vi "CRYMultimeter.vi"(0 "Device In":u32, 1 "Signal Path":i32(ring) caption="信号通道" items=["Left", "Right"], 2 "Mode":i32(slide), 3 "Time(sec)":dbl=5.0 caption="时间(秒)" min=0.05 max=10.0 step=0.05 format="%.0p", 4 "Avg.Time(sec)":dbl=1.0 caption="平均时间(秒)" min=0.05 max=1000.0 step=0.05 format="%.0p", 7 "Calibration in":string, 8 "Lin/Exp":i32(slide), 9 "Hardware in":string, 10 "Manual":bool=TRUE, 11 "Execution control":T3={"interactive"=TRUE, "displayed"=TRUE, "in a seq"=FALSE}, 13 "Cancel":bool) -> (6 "VMax In":dbl=1.0 min=0.1 max=10.0 step=0.01 format="%.3f", 12 "Canceled?":bool, 14 "InputLevel Out":T2, 15 "dB":cluster{dbl, dbl}(slide)={-inf, 99.22598823705182} scale=-70.01029995663981..19.989700043360187, 16 "Channel In":u16, 17 "Record time out":dbl format="%.2f", 18 "Averages out":i32, 19 "Overload":bool)   [LabVIEW 2013]
uses:
  Typedef Control/CRYData Cluster.ctl
  Typedef Control/CRYHardware Channel Info.ctl
  <vilib>/Analysis/baseanly.llb/Mean (DBL).vi
  <vilib>/Analysis/baseanly.llb/Real Dot Product.vi
  SubVI/CRYMisc vis settings global.vi
  Calibration/SubVI/CRYCal Global.vi
  Limits/CRYLimit edit global.vi
  CRYMainGlobal.vi
  Task Sequence/CRYProject Run Control Global.vi
  <vilib>/Analysis/NI_AALPro.lvlib
  <vilib>/Analysis/NI_AALBase.lvlib
  CRYSound.dll
panel:
  out "WWWW 2":dbl[](array[numeric])
  out "WWWW":dbl[](array[numeric])
  out "Corr Curve":T1={"Name"="", "Curve"=[], "X data"=1, "Y data"=1, "Z data"=1, "X axis"=0, "Y axis"=1, "Z axis"=1, "X unit"="Hz", "Y unit"="", "Z unit"="deg.", "X dB ref"=1.0, "Y dB ref"=1.0, "Z dB ref"=1.0, "single val"=FALSE, "protected"=FALSE, "display X"=TRUE, "display Y"=TRUE, "display Z"=TRUE, "Test Info"="", "Step No."=0, "Plot Settings"={"Color"=0, "Interpolation"=0, "Point Style"=0, "Line Style"=0, "Point Color"=0, "Line Width"=0, "Bar Plot Style"=0, "Fill To"=0}, "AutoProtect"=FALSE} {"Z data" items=["dB", "Lin"]; "X data" items=["dB", "Lin"]; "Y data" items=["dB", "Lin"]; "Z dB ref" format="%.1f"; "Z axis" items=["Log", "Lin"]; "X dB ref" format="%.1f"; "X axis" items=["Log", "Lin"]; "Y axis" items=["Log", "Lin"]; "Y dB ref" format="%.1f"; "Curve"."z" format="%.2f"; "Curve"."y" format="%.2f"; "Curve"."x" format="%.2f"}
  out "Waveform Graph":dbl[][](graph)
  out "y(n-1)":dbl
  in  "Buf Cnt":i32
  in  "isMain":bool
  in  "Rcv Idx":u16
  in  "start_flg":u8
  in  "ASIO_Inited":bool
  out "Asio OCI":u32
  in  "Remain Data":i32[](array[numeric])
  in  "Device Name":string
  in  "Audio Driver":u16
  out "Load Test":bool
  out "Set Configure":bool
  out "Configure Data":string
  out "Lower Str":bool
  out "Upper Str":bool
  out "initialized array":i32[](array[numeric])
  out "Menu":bool=TRUE
  out "StateOut":bool=TRUE
  out "VI nID":i32
  out "Title nID":i32
  out "User Avg.Time(sec)":dbl
  out "return type":u32
  out "multimeter setup Out":string="%#_6p"
  out "nBufferUse":u32
  out "RealTime":u32
  out "OverHead":u8
  in  "taskID":u32
  out "InputLevel":dbl caption="输入电平" step=1.0 format="%.3p"
  in  "Continue":bool
  out "AveString":bool
  in  "Start":bool
  in  "Lower limit":cluster{dbl, dbl}(slide)={100.0, 4.285714285714286} caption="Upper limit" scale=-70.01029995663981..19.989700043360187
  out "unit 2":string="dB"
  out "Averaging":bool caption="平均"
  out "Input":bool caption="输入"
  in  "Apply Correction":bool caption="修正"
  in  "Weighting":i32(ring) caption="加权" items=["None", "A", "B", "C"]
  out "Elapsed Time":dbl=50.0 caption="经过时间" min=0.05 max=100000.0 step=0.05 format="%.2p"
  in  "Time Weighting":i32(ring) caption="时间计权" items=["Fast", "Slow", "User"]
  in  "Level":i32(slide) caption="weighting"
  in  "Bits":u32=16
  in  "Sampling rate":u32=44100
  in  "Channels":u8=2
  in  "OK":bool
  in  "Limits On":bool caption="显示上下限"
  out "Buffer Use %":i32
  out "Verdict":bool=TRUE
  in  "AC/DC":i32(slide)
  out "dB ref.":dbl=1.0 format="%.2f"
  out "Sens":dbl=1.0 format="%.2f"
  out "unit":string="V"
  in  "close at end":bool
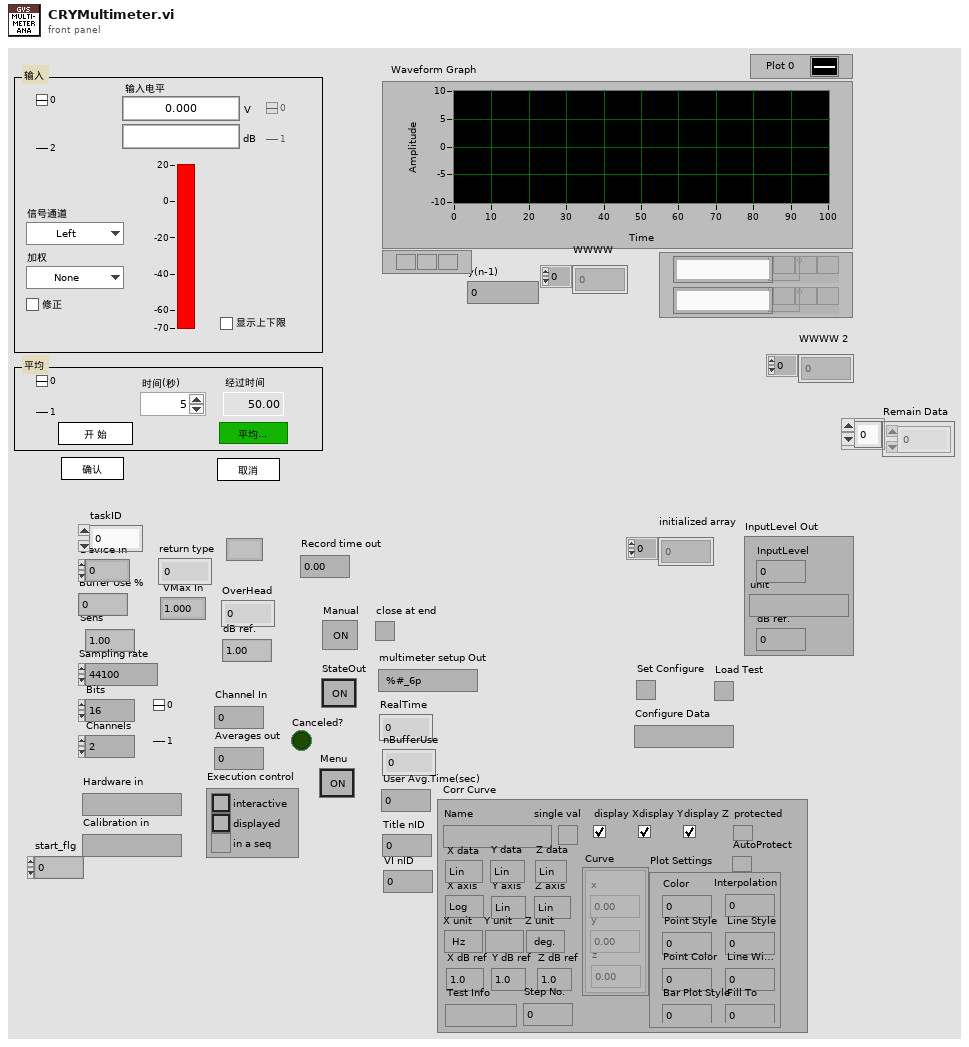
[diagram p1: front panel]
types:
  T1 = typedef "CRYData Cluster.ctl" = cluster{"Name":string, "Curve":cluster{"x":dbl, "y":dbl, "z":dbl}[], "X data":u16, "Y data":u16, "Z data":u16, "X axis":u16, "Y axis":u16, "Z axis":u16, "X unit":string, "Y unit":string, "Z unit":string, "X dB ref":dbl, "Y dB ref":dbl, "Z dB ref":dbl, "single val":bool, "protected":bool, "display X":bool, "display Y":bool, "display Z":bool, "Test Info":string, "Step No.":i32, "Plot Settings":cluster{"Color":u32, "Interpolation":u8, "Point Style":u8, "Line Style":u8, "Point Color":u32, "Line Width":u8, "Bar Plot Style":u8, "Fill To":i16}, "AutoProtect":bool}
  T2 = cluster{"InputLevel":dbl, "unit":string, "dB ref.":dbl}
  T3 = cluster{"interactive":bool, "displayed":bool, "in a seq":bool}
  T4 = cluster{"Start":bool, "Continue":bool, "OK":bool, "Cancel":bool, "Mode":i32, "Level":i32, "Channel":i32, "Weighting":i32, "Apply Correction":bool, "Limits On":bool, "Lin/Exp":i32, "Time Weighting":i32, "Time(sec)":dbl, "Avg.Time(sec)":dbl}
  T5 = typedef "CRYCalibration All Cluster.ctl" = cluster{"Calibration 2D":T6[], "Help":string, "Tab Value":i32, "Input Signal Type":string, "Output Signal Type":string}
  T6 = typedef "CRYCalibration 2DCluster.ctl" = cluster{"Calibration":T7, "Corr Curve":T1, "EQ Curve":T1, "Sens Curve":T1}
  T7 = typedef "CRYCalibration Cluster.ctl" = cluster{"Calibration Step Name":string, "Device":string, "Correction Curve Name":string, "Equalization Curve Name":string, "Sensitivity Curve Name":string, "Corr Folder and File":string, "EQ Folder and File":string, "Sens Folder and File":string, "Corr Step size":u16, "EQ Step size":u16, "Input":bool, "Last Cal Date (sec)":timestamp, "Cha Name":string, "Corr Curve Found":bool, "EQ Curve Found":bool, "Sens Curve Found":bool, "Signal Type":string, "Calibrated Device":string, "Hz":u32}
  T8 = typedef "CRYMultimeter.ctl" = cluster{"Ave/Max/Min":i32, "Level":i32, "Channel":i32, "Signal Type":string, "Weighting":string, "Applay Correction":bool, "lin/exp avg":u16, "rec time (sec)":dbl, "Average Time (Sec)":dbl, "Lin Display Prefs":string, "dB Display Prefs":string, "Time Weighting":u16, "Display":u16}
  T9 = typedef "CRYHardware Channel Info.ctl" = cluster{"ID":i32, "Name":string, "Digital":bool, "Input":bool, "Device Name":string, "Hardware Ch ID":u8, "Vmax (V)":dbl, "Latency (samples)":dbl, "Sampling Rate (Hz)":u32, "Bit Depth":u32, "Anti-aliasing Factor (%fs)":sgl, "DAQmx Channel":tag, "term config":i32, "Coupling":i32, "IEPE en":bool, "ASIOChannel Name":string, "Audio Driver":u16, "ASIOChannel Index":u8}
  T10 = typedef "LVPositionTypeDef.ctl" = cluster{"Left":i32, "Top":i32}
  T11 = cluster{"acquire":bool, "halt acq":bool, "n avgd":i32, "avg. complete":i32, "buffers":i32, "cal factor1":dbl, "cal factor2":dbl, "cal factor3":dbl, "update":bool, "Avg.weighting":dbl[], "Time Weighting":i32, "Avg.Time(sec)":dbl, "Continue":bool, "Mode":i32, "Level":i32, "Channel":i32, "rms max":dbl, "rms min":dbl, "avg. hold":dbl, "update ch":bool, "peak max":dbl, "peak min":dbl, "Weighting Curve":T1}
  T12 = cluster{"Start":bool, "Continue":bool, "OK":bool, "Cancel":bool, "Mode":i32, "Level":i32, "Signal Path":i32, "Weighting":i32, "Apply Correction":bool, "Limits On":bool, "Lin/Exp":i32, "Time Weighting":i32, "Time(sec)":dbl, "Avg.Time(sec)":dbl}
  T13 = cluster{"Rcv Idx":i32, "Chn Idx":i32, "Data":i32[], "bufCount":i32}[]
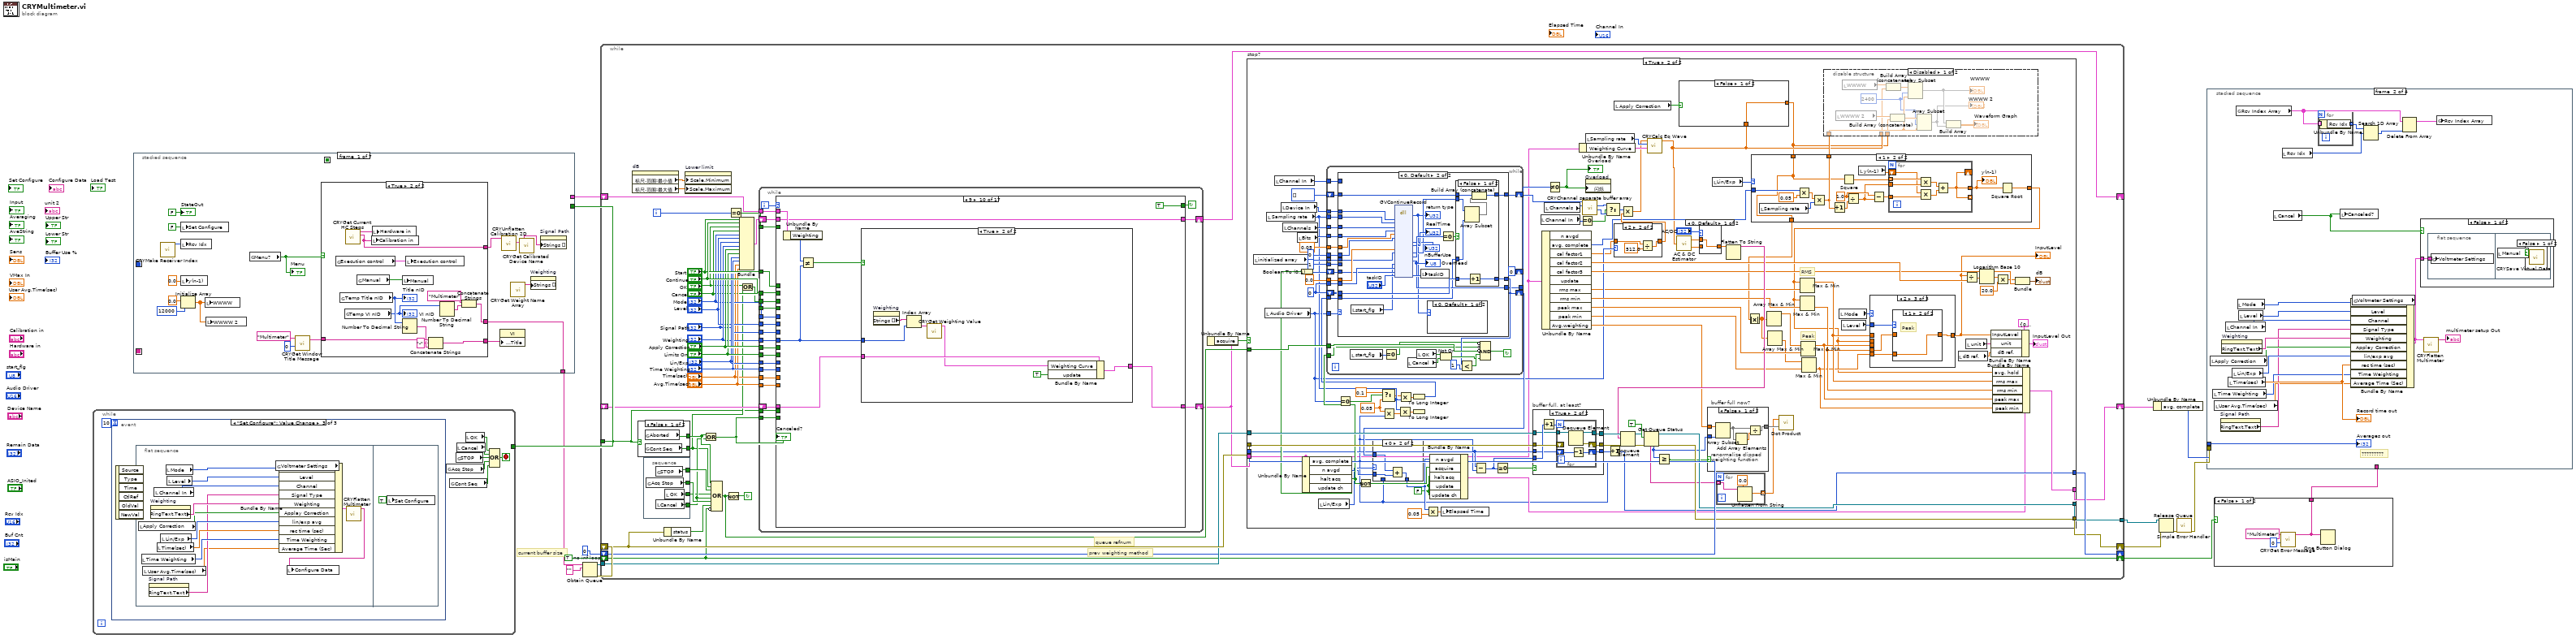
[diagram p0: block diagram]
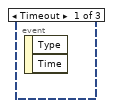
[diagram p2: hidden frame]
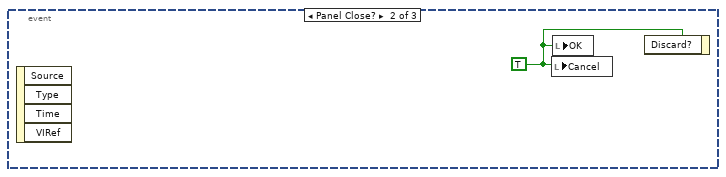
[diagram p3: hidden frame]
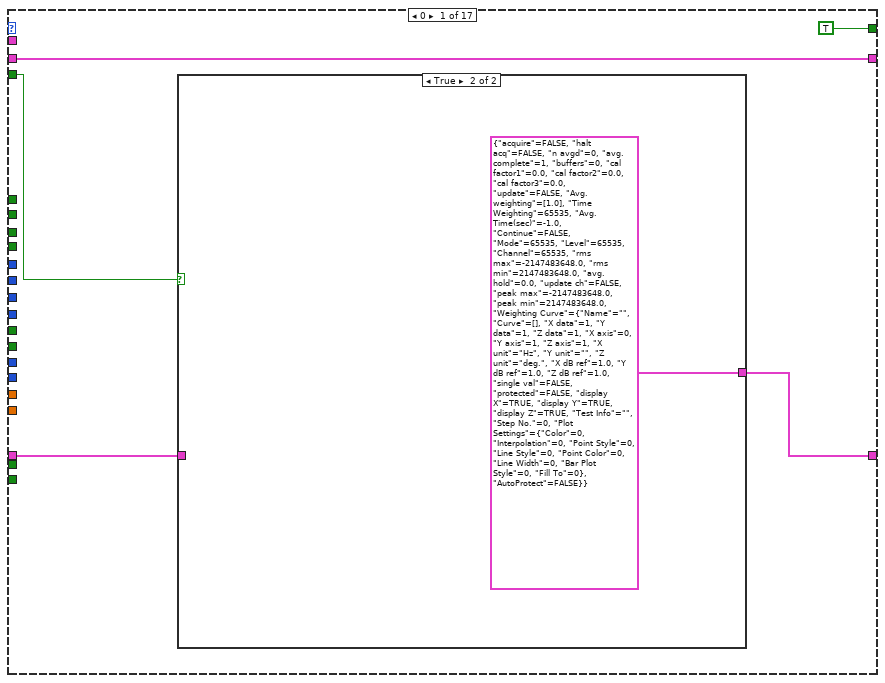
[diagram p4: hidden frame]
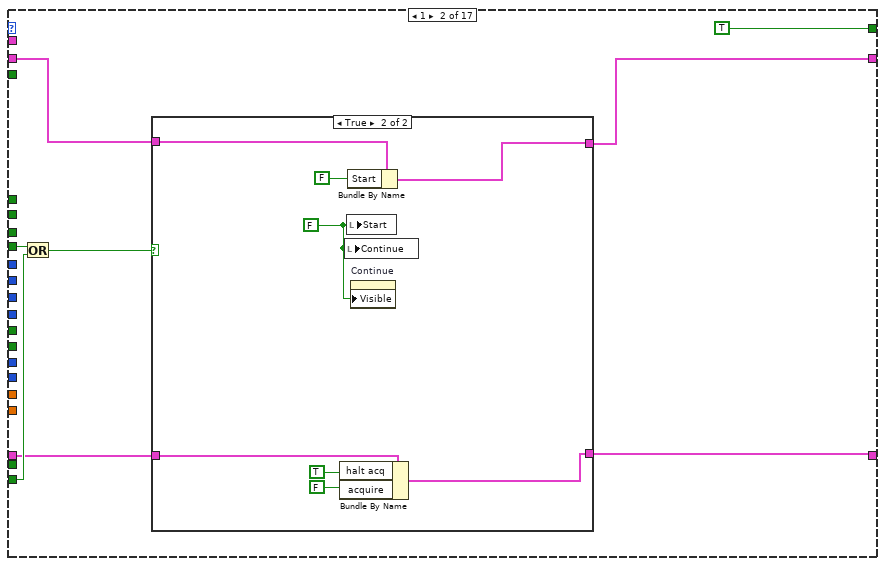
[diagram p6: hidden frame]
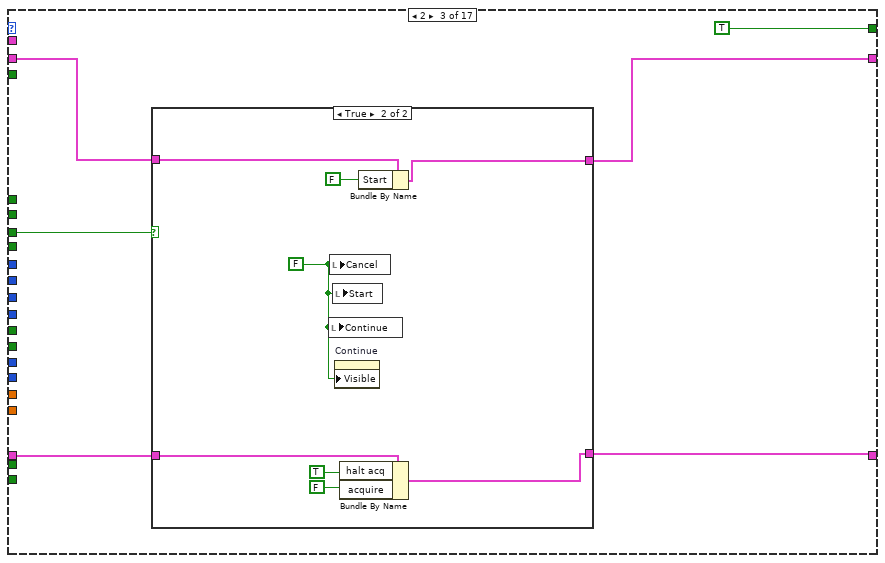
[diagram p8: hidden frame]
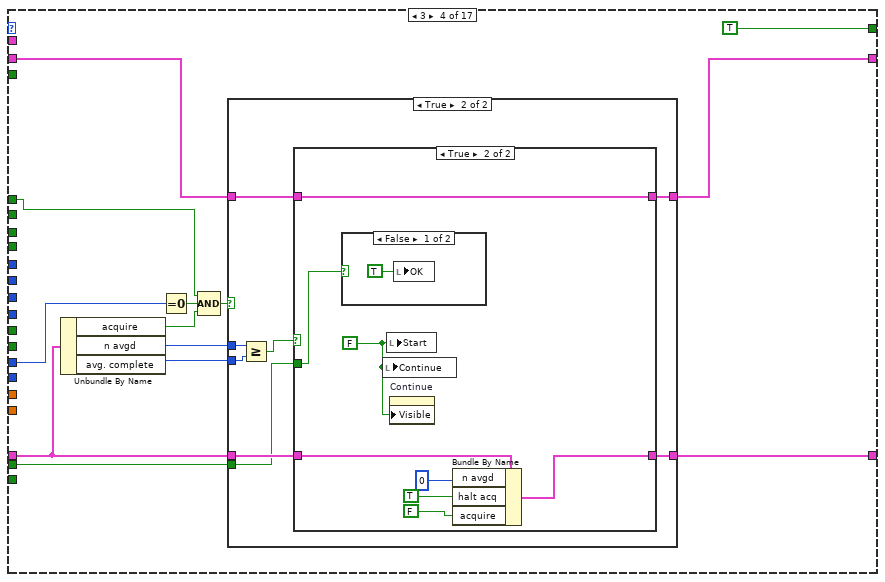
[diagram p10: hidden frame]
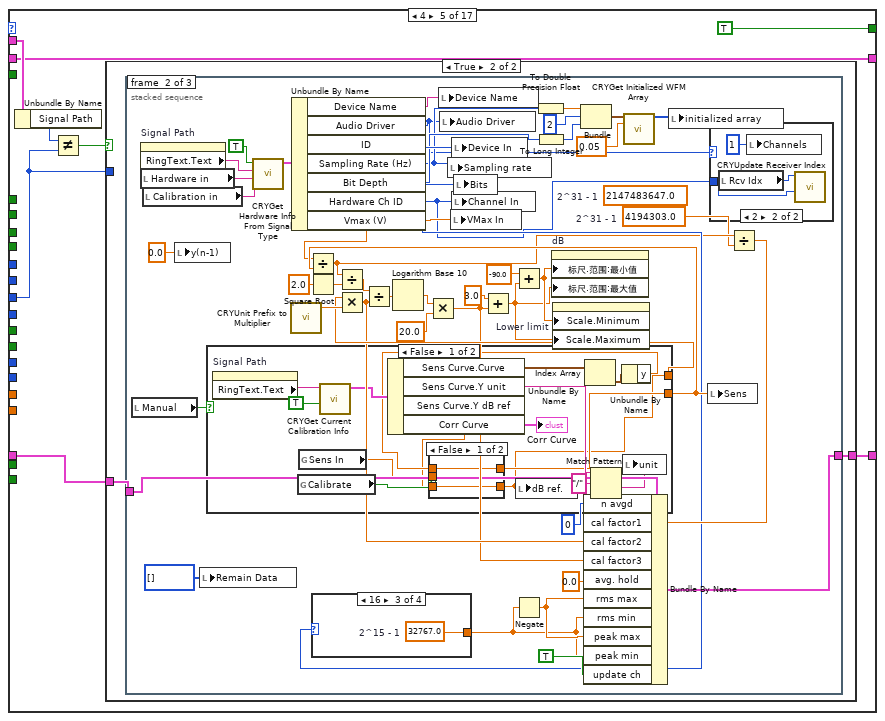
[diagram p14: hidden frame]
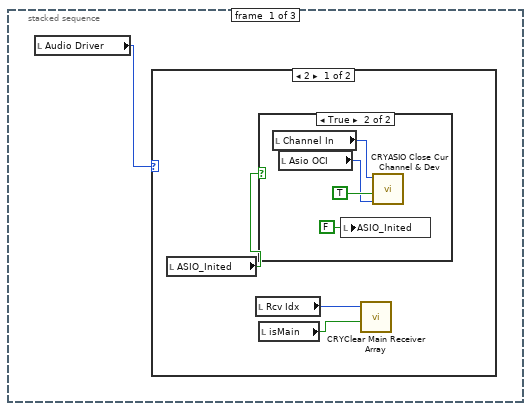
[diagram p16: hidden frame]
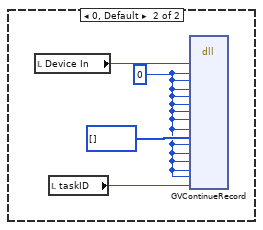
[diagram p18: hidden frame]
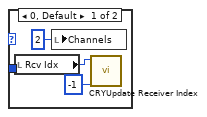
[diagram p19: hidden frame]
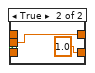
[diagram p20: hidden frame]
diagram:
  w15 = TRUE  # no inf loop
  # "current buffer size"
  n1 = stacked-sequence {
    seq-local: [_ w68 _ _ _ _ _] -> [_ _ _ w83 _ _ _]
    seq-local: [_ w53 _ _ _ _ _] -> [_ _ _ w84 _ _ _]
    seq-local: [_ _ w72 _ _ _ _] -> [_ _ _ _ _ _ _]
    tunnel: [_ _ w73 _ _ _ _] -> w2
    tunnel: [_ _ _ _ _ _ T4 {"Start"=FALSE, "Continue"=FALSE, "OK"=FALSE, "Cancel"=FALSE, "Mode"=-1, "Level"=0, "Channel"=-1, "Weighting"=-1, "Apply Correction"=FALSE, "Limits On"=FALSE, "Lin/Exp"=-1, "Time Weighting"=0, "Time(sec)"=-1.0, "Avg.Time(sec)"=0.05} ("cluster")] -> w7
    tunnel: [w25 _ _ _ _ _ _] -> w1
    frame #0 {
      n2 = call "CRYMake Receiver Index.vi"() -> ("Receiver_Index"=w21:i32)  [unwired: 11 in]
      n3 = local write "Set Configure"(FALSE ("Set Configure")) -> ()
      n4 = local write "Rcv Idx"(w21) -> ()
      n5 = local write "y(n-1)"(0.0) -> ()
      n6 = Initialize Array(0.0 ("element"), 12000 ("dimension size")) -> (w17:dbl[])
      n7 = local write "WWWW"(w17) -> ()
      n8 = local write "WWWW 2"(w17) -> ()
      n9 = global read "CRYMisc vis settings global.vi" "Menu?"() -> (w32:bool)
      "Menu" <- w32
      n10 = call "CRYGet Window Title Message.vi"("No"=0 ("Error No"), "Kind"="Multimeter") -> ("Multibyte String"=w28:string)  [unwired: 4 in, 5 out]
      n11 = case shown="True" w32 {
        tunnel: [w37 w48] -> w31
        tunnel: w28 -> [w37 w47]
        tunnel: ["Multimeter" ("名称（未命名）") w40] -> w25
        tunnel: [w35 w38] -> w22
        frame False {
          # "for Sequence Run"
          n12 = control-ref of="This VI"() -> (w34:refnum<vi>)
          n13 = call "CRYSet Multimeter Front Panel.vi"("Vi Ref in"=w34) -> ()  [unwired: 10 in, 1 out]
          n14 = local read "Calibration in"() -> (w35:string)
        }
        frame True {
          n15 = global read "CRYMisc vis settings global.vi" "Execution control"() -> (w46:T3)
          n16 = global read "CRYMisc vis settings global.vi" "Temp Title nID"() -> (w49:i32)
          "Title nID" <- w49
          n17 = global read "CRYMisc vis settings global.vi" "Temp VI nID"() -> (w43:i32)
          "VI nID" <- w43
          n18 = call "CRYGet Current HC Steps.vi"() -> ("Calibration setup flattened Out"=w38:string, "Hardware setup flattened Out"=w39:string)  [unwired: 10 out]
          n19 = global read "CRYMisc vis settings global.vi" "Manual"() -> (w50:bool)
          n20 = local write "Calibration in"(w38) -> ()
          n21 = local write "Hardware in"(w39) -> ()
          n22 = local write "Manual"(w50) -> ()
          n23 = Number To Decimal String(number=w49) -> (decimal integer string=w45:string)  [unwired: 1 in]
          n24 = local write "Execution control"(w46) -> ()
          n25 = Concatenate Strings(w47, "-" ("string"), w45) -> (w48:string)
          n26 = Number To Decimal String(number=w43) -> (decimal integer string=w42:string)  [unwired: 1 in]
          n27 = Concatenate Strings("Multimeter" ("名称（未命名）"), w42) -> (w40:string)
        }
      }
      n28 = property class="VI"("Front Panel.Title"=w31) -> ()  [unwired: 2 in, 2 out]
      n29 = call "CRYUnflatten Calibration 2D.vi"("Flattened Calibration"=w22) -> ("Calibration Step Out"=w23:T5)  [unwired: 8 in, 2 out]
      n30 = call "CRYGet Weight Name Array.vi"() -> ("Weighting Names"=w26:string[])  [unwired: 11 in]
      n31 = call "CRYGet Calibrated Device Name.vi"("Calibration"=w23) -> ("I_Signal Type Out"=w24:string[])  [unwired: 7 in, 7 out]
      n32 = property on="Weighting" class="Ring (strict)"("Strings []"=w26) -> ()  [unwired: 2 in, 2 out]
      n33 = property on="Signal Path" class="Ring (strict)"("Strings []"=w24) -> ()  [unwired: 2 in, 2 out]
      "StateOut" <- FALSE ("StateOut")
    }
    frame #1 {
      # "????????"
      n34 = global read "CRYMisc vis settings global.vi" "Voltmeter Settings"() -> (w71:T8)
      n35 = Unbundle By Name(w71) -> ("Ave/Max/Min"=w70:i32, "Level"=w69:i32, "Channel"=w68:i32, "Signal Type"=w53:string, "Weighting"=w58:string, "Applay Correction"=w67:bool, "lin/exp avg"=w66:u16, "rec time (sec)"=w65:dbl, "Time Weighting"=w64:u16, "Average Time (Sec)"=w51:dbl)
      n36 = local write "User Avg.Time(sec)"(w51) -> ()
      n37 = local write "Apply Correction"(w67) -> ()
      n38 = local write "Time Weighting"(w64) -> ()
      n39 = local write "Mode"(w70) -> ()
      n40 = local write "Channel In"(w68) -> ()
      n41 = local write "Time(sec)"(w65) -> ()
      n42 = local write "Level"(w69) -> ()
      n43 = local write "Lin/Exp"(w66) -> ()
      n44 = property on="Signal Path" class="Ring (strict)"() -> ("Strings []"=w52:string[])  [unwired: 2 in, 2 out]
      n45 = property on="Weighting" class="Ring (strict)"() -> ("Strings []"=w63:string[])  [unwired: 2 in, 2 out]
      n46 = Search 1D Array(1D array=w52, element=w53) -> (index of element=w56:i32)  [unwired: 1 out]
      n47 = Search 1D Array(1D array=w63, element=w58) -> (index of element=w60:i32)  [unwired: 1 out]
      n48 = Less Than 0?(x=w56) -> (x < 0?=w55:bool)
      n49 = Less Than 0?(x=w60) -> (x < 0?=w61:bool)
      n50 = Select(t=0 ("index of element"), s=w55, f=w56) -> (s? t:f=w57:i32)
      n51 = Select(t=0 ("index of element"), s=w61, f=w60) -> (s? t:f=w59:i32)
      n52 = property on="Signal Path" class="Ring (strict)"("Value"=w57) -> ()  [unwired: 2 in, 2 out]
      n53 = property on="Weighting" class="Ring (strict)"("Value"=w59) -> ()  [unwired: 2 in, 2 out]
    }
    frame #2 {
      n54 = Unbundle By Name("Execution control") -> ("in a seq"=w72:bool, "interactive"=w74:bool, "displayed"=w79:bool)
      n55 = property class="VI"() -> ("前面板窗口:打开"=w76:bool)  [unwired: 2 in, 2 out]
      n56 = Or(x=w74, y=w79) -> (x .or. y?=w77:bool)
      n57 = Not(x=w72) -> (.not. x?=w73:bool)
      n58 = Compound Arithmetic op=AND(w77, invert w76) -> (w75:bool)
      n59 = case shown="True" w77 {
        tunnel: w77 -> [_ w80]
        tunnel: w75 -> [_ _]
        frame False {
        }
        frame True {
          n60 = stacked-sequence {
            tunnel: w80 -> [w81 _]
            frame #0 {
              n61 = property class="VI"("前面板窗口:打开"=w81) -> ()  [unwired: 2 in, 2 out]
            }
            frame #1 {
              n62 = Wait (ms)(milliseconds to wait=u32 150) -> ()  [unwired: 1 out]
            }
          }
        }
      }
      n63 = local write "close at end"(w75) -> ()
    }
    frame #3 {
      n64 = case shown="True" "Manual" {
        tunnel: w84 -> [w87 _]
        tunnel: w83 -> [w86 _]
        frame False {
          n65 = stacked-sequence {
            tunnel: w87 -> [w93 _ _]
            tunnel: w86 -> [_ _ _]
            frame #0 {
              n66 = global read "CRYCal Global.vi" "Calibrate"() -> (w96:bool)
              n67 = local read "Calibration in"() -> (w94:string)
              n68 = local read "Hardware in"() -> (w95:string)
              n69 = case shown="True" w96 {
                tunnel: w93 -> [w113 _]
                tunnel: [w116 w131] -> w92
                tunnel: w95 -> [w115 w133]
                tunnel: w94 -> [w114 w132]
                tunnel: [w110 w130] -> w97
                frame False {
                  n70 = call "CRYGet Hardware Info From Signal Type.vi"("Calibration In"=w114, "Hardware In"=w115, "Signal Type"=w113, "In/Out?"=TRUE) -> ("Exist?"=w118:bool, "Channel Info Out"=w117:T9)  [unwired: 5 in, 1 out]
                  n71 = property on="Signal Path" class="Ring (strict)"() -> ("Strings []"=w112:string[])  [unwired: 2 in, 2 out]
                  n72 = case shown="False" w118 {
                    tunnel: w117 -> [_ w126]
                    tunnel: [w121 w126] -> w116
                    tunnel: w115 -> [w124 _]
                    tunnel: w114 -> [w123 _]
                    tunnel: w113 -> [_ w125]
                    tunnel: [w120 w125] -> w111
                    frame False {
                      w120 = "Direct In 1" ("Signal Type")
                      n73 = call "CRYGet Hardware Info From Signal Type.vi"("Calibration In"=w123, "Hardware In"=w124, "Signal Type"=w120, "In/Out?"=TRUE) -> ("Channel Info Out"=w121:T9)  [unwired: 5 in, 2 out]
                    }
                    frame True {
                    }
                  }
                  n74 = Search 1D Array(1D array=w112, element=w111) -> (index of element=w110:i32)  [unwired: 1 in]
                }
                frame True {
                  n75 = global read "CRYCal Global.vi" "Signal Type In"() -> (w130:u16)
                  n76 = property on="Signal Path" class="Ring (strict)"() -> ("Strings []"=w129:string[])  [unwired: 2 in, 2 out]
                  n77 = Index Array(array=w129, index=w130) -> (element=w127:string)
                  n78 = call "CRYGet Hardware Info From Signal Type.vi"("Calibration In"=w132, "Hardware In"=w133, "Signal Type"=w127, "In/Out?"=TRUE) -> ("Channel Info Out"=w131:T9)  [unwired: 5 in, 2 out]
                }
              }
              n79 = Unbundle By Name(w92) -> ("Device Name"=w91:string, "Audio Driver"=w90:u16, "ID"=w103:i32, "Vmax (V)"=w99:dbl, "Sampling Rate (Hz)"=w102:u32, "Bit Depth"=w101:u32, "Hardware Ch ID"=w88:u8)
              n80 = local write "Signal Path"(w97) -> ()
              n81 = local write "ASIO_Inited"(FALSE ("ASIO_Inited")) -> ()
              n82 = case shown="0, Default" w90 {
                tunnel: w88 -> [_ w107]
                frame 0, Default {
                  n83 = local read "Rcv Idx"() -> (w105:u16)
                  n84 = local write "Channels"(u8 2 ("Channels")) -> ()
                  n85 = call "CRYUpdate Receiver Index.vi"("Chn Idx"=-1, "Receiver_Index"=w105) -> ()  [unwired: 9 in]
                }
                frame 2 {
                  n86 = local read "Rcv Idx"() -> (w108:u16)
                  n87 = local write "Channels"(u8 1 ("Channels")) -> ()
                  n88 = call "CRYUpdate Receiver Index.vi"("Chn Idx"=w107, "Receiver_Index"=w108) -> ()  [unwired: 9 in]
                }
              }
              n89 = Select(t=1.0 ("Vmax (V)"), s=w96, f=w99) -> (s? t:f=w98:dbl)
              n90 = local write "Bits"(w101) -> ()
              n91 = local write "Sampling rate"(w102) -> ()
              n92 = local write "Device Name"(w91) -> ()
              n93 = local write "Channel In"(w88) -> ()
              n94 = local write "Audio Driver"(w90) -> ()
              n95 = local write "Device In"(w103) -> ()
              n96 = local write "VMax In"(w98) -> ()
            }
            frame #1 {
              n97 = property on="Signal Path" class="Ring (strict)"() -> ("RingText.Text"=w141:string)  [unwired: 2 in, 2 out]
              n98 = call "CRYGet Current Calibration Info.vi"("Is Input?"=TRUE, "Signal Type Name"=w141) -> ("Calibration All Cluster"=w140:T6)  [unwired: 9 out]
              n99 = Unbundle By Name(w140) -> ("Sens Curve.Curve"=w144:cluster{"x":dbl, "y":dbl, "z":dbl}[], "Sens Curve.Y unit"=w137:string, "Sens Curve.Y dB ref"=w136:dbl)
              n100 = Index Array(array=w144) -> (element=w143:cluster{"x":dbl, "y":dbl, "z":dbl})  [unwired: 1 in]
              n101 = Match Pattern(string=w137, regular expression="/" ("search char (-)")) -> (after substring=→"unit":string)  [unwired: 4 out]
              n102 = Unbundle By Name(w143) -> ("y"=w139:dbl)
              n103 = global read "CRYCal Global.vi" "Calibrate"() -> (w146:bool)
              n104 = case shown="False" w146 {
                tunnel: [w148 w149] -> w145
                tunnel: w139 -> [w148 _]
                tunnel: w136 -> [w147 _]
                tunnel: [w147 1.0 ("Y dB ref")] -> w134
                frame False {
                }
                frame True {
                  n105 = global read "CRYCal Global.vi" "Sens In"() -> (w149:dbl)
                }
              }
              "dB ref." <- w134
              n106 = local write "Sens"(w145) -> ()
            }
            frame #2 {
              # "??????????"
              n107 = global read "CRYLimit edit global.vi" "Limits On"() -> (w151:bool)
              n108 = local write "Limits On"(w151) -> ()
              n109 = case shown="True" w151 {
                frame False {
                }
                frame True {
                  n110 = global read "CRYLimit edit global.vi" "Lower Limit"() -> (w152:dbl)
                  n111 = global read "CRYLimit edit global.vi" "Upper Limit"() -> (w153:dbl)
                  n112 = Bundle("Upper Limit"=w153, "Lower Limit"=w152) -> (w154:cluster{"Upper Limit":dbl, "Lower Limit":dbl})  [unwired: 1 out]
                  n113 = local write "Lower limit"(w154) -> ()
                }
              }
            }
          }
        }
        frame True {
          w158 = 0 items=["Fast", "Slow", "User"] ("Time Weighting")
          w162 = 0 items=["Average", "Maximum", "Minimum"] ("Mode")
          w161 = 0 items=["Linear", "Exponential"] ("weighting")
          (unwired) T9[] [{"ID"=2, "Name"="Left", "Digital"=FALSE, "Input"=TRUE, "Device Name"="Card", "Hardware Ch ID"=0, "Vmax (V)"=10.0, "Latency (samples)"=67.0, "Sampling Rate (Hz)"=44100, "Bit Depth"=16, "Anti-aliasing Factor (%fs)"=44100.0, "DAQmx Channel"="", "term config"=0, "Coupling"=0, "IEPE en"=FALSE, "ASIOChannel Name"="", "Audio Driver"=0, "ASIOChannel Index"=0}, {"ID"=2, "Name"="Left", "Digital"=FALSE, "Input"=TRUE, "Device Name"="Card", "Hardware Ch ID"=1, "Vmax (V)"=10.0, "Latency (samples)"=67.0, "Sampling Rate (Hz)"=44100, "Bit Depth"=16, "Anti-aliasing Factor (%fs)"=44100.0, "DAQmx Channel"="", "term config"=0, "Coupling"=0, "IEPE en"=FALSE, "ASIOChannel Name"="", "Audio Driver"=0, "ASIOChannel Index"=0}] ("I_channel Info Out")
          w163 = 0 items=["Left", "Right"] ("Channel")
          n114 = local write "Apply Correction"(FALSE ("Apply\nCorrection")) -> ()
          n115 = local write "Time Weighting"(w158) -> ()
          n116 = local write "Avg.Time(sec)"(0.25 ("Avg.Time(sec)")) -> ()
          n117 = local write "Mode"(w162) -> ()
          n118 = local write "Channel In"(u16 0 ("Channel In")) -> ()
          n119 = local write "Time(sec)"(0.05 ("Time(sec)")) -> ()
          n120 = local write "Lin/Exp"(w161) -> ()
          n121 = local write "Signal Path"(w163) -> ()
          n122 = local write "Sampling rate"(u32 44100 ("Sampling rate")) -> ()
          n123 = local write "Device In"(u16 2 ("Device In")) -> ()
          n124 = local write "Bits"(16 ("Bits")) -> ()
          n125 = local write "User Avg.Time(sec)"(0.05 ("User Time")) -> ()
          n126 = local write "VMax In"(10.0 ("y")) -> ()
          n127 = local write "Channels"(u8 2 ("Channels")) -> ()
          n128 = property on="Signal Path" class="Ring (strict)"("Strings []"=string[] ["Left", "Right"]) -> ()  [unwired: 2 in, 2 out]
          n129 = local write "dB ref."(1.0 ("dB ref.")) -> ()
          n130 = local write "Sens"(1.0 ("Sens.")) -> ()
          n131 = local write "unit"("V" ("unit")) -> ()
        }
      }
    }
    frame #4 {
      w178 = TRUE ("Start")
      w175 = FALSE ("Visible")
      w179 = FALSE ("STOP")
      w180 = FALSE ("Limits On")
      n132 = disable-structure shown="禁用" {
        frame Disabled {
          n133 = property on="Elapsed Time" class="DigNum (strict)"() -> ("Position"=w184:T10)  [unwired: 2 in, 2 out]
          n134 = property on="Time(sec)" class="DigNum (strict)"() -> ("Position"=w185:T10)  [unwired: 2 in, 2 out]
          n135 = property on="Avg.Time(sec)" class="DigNum (strict)"("Position"=w184) -> ()  [unwired: 2 in, 2 out]
          n136 = property on="Time Weighting" class="Ring (strict)"("Position"=w185) -> ()  [unwired: 2 in, 2 out]
        }
        frame Enabled {
        }
      }
      n137 = local write "Limits On"(w180) -> ()
      n138 = local write "Continue"(w180) -> ()
      n139 = local write "Cancel"(w179) -> ()
      n140 = local write "Start"(w178) -> ()
      n141 = local write "OK"(w179) -> ()
      n142 = property on="Start" class="Bool (strict)"("Visible"=w178) -> ()  [unwired: 2 in, 2 out]
      n143 = property on="Continue" class="Bool (strict)"("Visible"=w180) -> ()  [unwired: 2 in, 2 out]
      n144 = global write "CRYMainGlobal.vi" "STOP"(w179) -> ()
      n145 = local write "Elapsed Time"(0.0 ("Elapsed Time")) -> ()
      n146 = global write "CRYLimit edit global.vi" "Limits On"(w175) -> ()
      n147 = property on="Verdict" class="Bool (strict)"("可见"=w175) -> ()  [unwired: 2 in, 2 out]
      n148 = call "CRYGet Error Message.vi"("Error No"=0, "Kind"="Multimeter Sub") -> ("Unicode Message Sub"=w174:string[])  [unwired: 4 in, 5 out]
      n149 = property on="Lower limit" class="Slide (strict)"("Visible"=w175) -> ()  [unwired: 2 in, 2 out]
      n150 = for {
        tunnel: w174 -> [w183] mode=indexing
        tunnel: [w182] -> w173 mode=indexing
        n151 = call "CRYConvert Unicode to ASCII.vi"("Unicode"=w183) -> ("ASCII"=w182:string)  [unwired: 4 in]
      }
      n152 = property on="Upper Str" class="Bool (strict)"("Visible"=w175) -> ()  [unwired: 2 in, 2 out]
      n153 = property on="Start" class="Bool (strict)"("Strings [4]"=w173) -> ()  [unwired: 2 in, 2 out]
      n154 = property on="Lower Str" class="Bool (strict)"("Visible"=w175) -> ()  [unwired: 2 in, 2 out]
    }
    frame #5 {
      n155 = local read "Sampling rate"() -> (w192:u32)
      n156 = local read "Bits"() -> (w190:u32)
      n157 = To Double Precision Float(number=w192) -> (double precision float=w191:dbl)
      n158 = To Long Integer(number=w190) -> (32bit integer=w189:i32)
      n159 = Bundle(w191, "32bit integer"=2, w189) -> (w187:cluster{dbl, "32bit integer":i32, i32})  [unwired: 1 in]
      n160 = call "CRYGet Initialized WFM Array.vi"("Sound Format"=w187, "Time(s)"=0.05) -> ("initialized array"=→"initialized array":i32[])  [unwired: 8 in, 5 out]
    }
    frame #6 {
      w200 = 10.0 ("y")
      w199 = 0.05 ("y")
      w207 = 10.0 ("y")
      w208 = 0.05 ("y")
      n161 = local write "start_flg"(u8 1 ("start_flg")) -> ()
      n162 = local read "User Avg.Time(sec)"() -> (w197:dbl)
      n163 = local read "Time(sec)"() -> (w203:dbl)
      n164 = Greater?(x=w208, y=w203) -> (0:w209:bool)
      n165 = Greater?(x=w199, y=w197) -> (0:w198:bool)
      n166 = local write "Load Test"(TRUE ("Load Test")) -> ()
      n167 = Select(t=w208, s=w209, f=w203) -> (s? t:f=w205:dbl)
      n168 = Select(t=w199, s=w198, f=w197) -> (s? t:f=w202:dbl)
      n169 = Less?(x=w207, y=w205) -> (x < y?=w206:bool)
      n170 = Less?(x=w200, y=w202) -> (x < y?=w201:bool)
      n171 = Select(t=w207, s=w206, f=w205) -> (s? t:f=w204:dbl)
      n172 = Select(t=w200, s=w201, f=w202) -> (s? t:f=w196:dbl)
      n173 = local write "User Avg.Time(sec)"(w196) -> ()
      n174 = local write "Time(sec)"(w204) -> ()
    }
  }
  n175 = while {
    tunnel: w2 -> [_]
    stop <- w215 stop-if-true
    n176 = event shown="[2] \"Set Configure\": Value Change" {
      selector: _ -> [_ _ _]
      dyn-events: _ -> [_ _ _]
      timeout: 10 -> [_ _ _]
      event Timeout {
        n177 = event-data() -> ()  [unwired: 3 out]
      }
      event Panel Close? {
        w218 = TRUE ("Discard?")
        n178 = event-data() -> ()  [unwired: 5 out]
        n179 = local write "Cancel"(w218) -> ()
        n180 = local write "OK"(w218) -> ()
        n181 = event-data("Discard?"=w218) -> ()  [unwired: 1 in, 1 out]
      }
      event "Set Configure": Value Change {
        n182 = event-data() -> ()  [unwired: 7 out]
        n183 = flat-sequence {
          frame #0 {
            n184 = local read "Apply Correction"() -> (w226:bool)
            n185 = local read "Time Weighting"() -> (w224:i32)
            n186 = local read "User Avg.Time(sec)"() -> (w221:dbl)
            n187 = property on="Signal Path" class="Ring (strict)"() -> ("RingText.Text"=w223:string)  [unwired: 2 in, 2 out]
            n188 = property on="Weighting" class="Ring (strict)"() -> ("RingText.Text"=w227:string)  [unwired: 2 in, 2 out]
            n189 = local read "Channel In"() -> (w229:u16)
            n190 = local read "Time(sec)"() -> (w230:dbl)
            n191 = local read "Lin/Exp"() -> (w225:i32)
            n192 = local read "Mode"() -> (w228:i32)
            n193 = local read "Level"() -> (w222:i32)
            n194 = global read "CRYMisc vis settings global.vi" "Voltmeter Settings"() -> (w219:T8)
            n195 = Bundle By Name(cluster=w219, "Ave/Max/Min"=w228, "Level"=w222, "Channel"=w229, "Signal Type"=w223, "Weighting"=w227, "Applay Correction"=w226, "lin/exp avg"=w225, "rec time (sec)"=w230, "Time Weighting"=w224, "Average Time (Sec)"=w221) -> (w231:T8)
            n196 = call "CRYFlatten Multimeter.vi"("Voltmeter Settings"=w231) -> ("Flat Voltmeter setup"=w220:string)  [unwired: 10 out]
            n197 = local write "Configure Data"(w220) -> ()
          }
          frame #1 {
            n198 = local write "Set Configure"(TRUE ("Set Configure")) -> ()
          }
        }
      }
    }
    n199 = global read "CRYMainGlobal.vi" "Acq Stop"() -> (w212:bool)
    n200 = global read "CRYProject Run Control Global.vi" "Cont Seq"() -> (w211:bool)
    n201 = global read "CRYMainGlobal.vi" "STOP"() -> (w214:bool)
    n202 = local read "Cancel"() -> (w216:bool)
    n203 = local read "OK"() -> (w213:bool)
    n204 = Compound Arithmetic op=OR(w213, w216, w214, w212, w211) -> (w215:bool)
  }
  n205 = Obtain Queue(name (unnamed)=w1, element data type="") -> (queue out=w13:refnum<queue>, error out=w14:errorcluster)  [unwired: 3 in, 1 out]
  n206 = while {
    tunnel: w2 -> [w236]
    shift-left: w15 -> [w265]
    shift-right: [w265] -> w5
    shift-left: w14 -> [w274]
    shift-right: [w275] -> w10
    shift-left: 0 -> [w267]
    shift-right: [w276] -> _
    tunnel: w13 -> [w273]
    tunnel: [w264] -> w11
    shift-right: [w244] -> w4
    shift-left: _ -> [w248]
    shift-right: [w245] -> _
    shift-left: w7 -> [w249]
    i -> [w233]
    stop <- w234 continue-if-true
    # "prev weighting method"
    # "queue refnum"
    n207 = property on="dB" class="Slide (strict)"() -> ("标尺.范围:最小值"=w262:dbl, "标尺.范围:最大值"=w263:dbl)  [unwired: 2 in, 2 out]
    n208 = case shown="False" w236 {
      tunnel: [w1148 w1151] -> w269
      tunnel: [w1149 w1150] -> w238
      frame False {
        n209 = global read "CRYProject Run Control Global.vi" "Aborted"() -> (w1148:bool)
        n210 = global read "CRYProject Run Control Global.vi" "Cont Seq"() -> (w1149:bool)
      }
      frame True {
        n211 = global read "CRYProject Run Control Global.vi" "Cancel fsw"() -> (w1151:bool)
        n212 = global read "CRYProject Run Control Global.vi" "OK fsw"() -> (w1150:bool)
      }
    }
    n213 = stacked-sequence {
      tunnel: [w1152] -> w268
      tunnel: [w1153] -> w272
      tunnel: [w1155] -> w270
      tunnel: [w1154] -> w266
      frame #0 {
        n214 = global read "CRYMainGlobal.vi" "Acq Stop"() -> (w1154:bool)
        n215 = global read "CRYMainGlobal.vi" "STOP"() -> (w1155:bool)
        n216 = local read "Cancel"() -> (w1152:bool)
        n217 = local read "OK"() -> (w1153:bool)
      }
    }
    n218 = Unbundle By Name(w274) -> ("status"=w271:bool)
    n219 = property on="Lower limit" class="Slide (strict)"("Scale.Minimum"=w262, "Scale.Maximum"=w263) -> ()  [unwired: 2 in, 2 out]
    n220 = Or(x=w269, y=w268) -> (x .or. y?=w240:bool)
    "Canceled?" <- w240
    n221 = Compound Arithmetic op=OR(w269, w238, w270, w266, w268, w272, w271, invert w265) -> (w243:bool)
    n222 = Not(x=w243) -> (.not. x?=w234:bool)
    n223 = Equal To 0?(x=w233) -> (x = 0?=w251:bool)
    n224 = Bundle("Start"="Start", "Continue"="Continue", "OK"="OK", "Cancel"="Cancel", "Mode"="Mode", "Level"="Level", "Signal Path"="Signal Path", "Weighting"="Weighting", "Apply Correction"="Apply Correction", "Limits On"="Limits On", "Lin/Exp"="Lin/Exp", "Time Weighting"="Time Weighting", "Time(sec)"="Time(sec)", "Avg.Time(sec)"="Avg.Time(sec)") -> (w250:T12)  [unwired: 1 out]
    n225 = Or(x="OK", y=w238) -> (x .or. y?=w237:bool)
    n226 = while {
      shift-right: [w298] -> w245
      shift-left: w250 -> [w299]
      tunnel: w249 -> [w300]
      tunnel: w251 -> [w297]
      tunnel: "Mode" -> [w296]
      tunnel: "Signal Path" -> [w295]
      tunnel: "Level" -> [w294]
      tunnel: "Weighting" -> [w293]
      tunnel: "Lin/Exp" -> [w292]
      tunnel: "Time Weighting" -> [w291]
      tunnel: "Limits On" -> [w290]
      tunnel: "Apply Correction" -> [w289]
      shift-right: [w287] -> w235
      shift-left: w248 -> [w286]
      tunnel: "Start" -> [w285]
      tunnel: "Continue" -> [w284]
      tunnel: "Avg.Time(sec)" -> [w283]
      tunnel: "Time(sec)" -> [w282]
      tunnel: "Cancel" -> [w281]
      tunnel: w240 -> [w280]
      tunnel: w237 -> [w279]
      tunnel: w236 -> [w278]
      i -> [w277]
      stop <- w288 continue-if-true
      n227 = case shown="9" w277 {
        tunnel: w300 -> [_ _ _ _ w382 w494 w501 w512 w522 w571 w585 w592 w600 w624 w651 w679 w800]
        tunnel: w299 -> [w302 w309 w327 w345 w378 w493 w502 w509 w521 w569 w582 w588 w598 w620 w646 w673 w803]
        tunnel: [w302 w308 w326 w344 w378 w493 w502 w509 w521 w569 w582 w588 w598 w620 w646 w672 w803] -> w298
        tunnel: w297 -> [w304 _ _ _ _ _ _ _ _ _ _ _ _ _ _ _ w789]
        tunnel: w296 -> [_ _ _ _ _ _ w498 _ _ _ _ _ _ _ _ _ _]
        tunnel: w295 -> [_ _ _ _ w377 _ _ _ _ _ _ _ _ _ _ _ _]
        tunnel: w294 -> [_ _ _ _ _ _ _ w511 _ _ _ _ _ _ _ _ _]
        tunnel: w293 -> [_ _ _ _ _ _ _ _ _ w565 _ _ _ _ _ _ _]
        tunnel: w292 -> [_ _ _ w353 _ _ _ _ w519 _ _ _ _ w617 w642 w675 w788]
        tunnel: w291 -> [_ _ _ _ _ _ _ _ w516 _ _ _ w595 _ w649 _ _]
        tunnel: w290 -> [_ _ _ _ _ _ _ _ _ _ _ w590 _ _ _ _ _]
        tunnel: w289 -> [_ _ _ _ _ _ _ _ _ _ w584 _ _ _ _ _ _]
        tunnel: [TRUE ("Is Input?") TRUE ("Is Input?") TRUE ("Is Input?") TRUE ("Is Input?") TRUE ("Is Input?") TRUE ("Visible") TRUE TRUE TRUE ("Is Input?") TRUE ("Is Input?") TRUE ("Is Input?") TRUE ("Is Input?") TRUE ("Is Input?") TRUE ("Is Input?") TRUE ("Is Input?") TRUE FALSE ("Is Input?")] -> w288
        tunnel: [w305 w311 w330 w354 w380 w490 w496 w508 w517 w566 w581 w587 w597 w618 w643 w676 w790] -> w287
        tunnel: w286 -> [w303 w310 w328 w352 w381 w490 w496 w508 w518 w567 w581 w587 w597 w619 w644 w677 w791]
        tunnel: w285 -> [_ _ _ w343 _ _ _ _ _ _ _ _ _ _ _ w671 _]
        tunnel: w284 -> [_ _ _ _ _ w491 _ _ _ _ _ _ _ _ _ w670 _]
        tunnel: w283 -> [_ _ _ _ _ _ _ _ _ _ _ _ _ _ w645 w667 w793]
        tunnel: w282 -> [_ _ _ _ _ _ _ _ w514 _ _ _ _ w622 _ w669 w799]
        tunnel: w281 -> [_ w315 _ _ _ _ _ _ _ _ _ _ _ _ _ _ _]
        tunnel: w280 -> [_ w314 _ _ _ _ _ _ _ _ _ _ _ _ _ _ _]
        tunnel: w279 -> [_ _ w329 _ _ _ _ _ _ _ _ _ _ _ _ _ _]
        tunnel: w278 -> [_ _ _ w346 _ _ _ _ _ _ _ _ _ _ _ _ _]
        frame 0 {
          n228 = case shown="True" w304 {
            tunnel: [w306 T11 {"acquire"=FALSE, "halt acq"=FALSE, "n avgd"=0, "avg. complete"=1, "buffers"=0, "cal factor1"=0.0, "cal factor2"=0.0, "cal factor3"=0.0, "update"=FALSE, "Avg.weighting"=[1.0], "Time Weighting"=65535, "Avg.Time(sec)"=-1.0, "Continue"=FALSE, "Mode"=65535, "Level"=65535, "Channel"=65535, "rms max"=-2147483648.0, "rms min"=2147483648.0, "avg. hold"=0.0, "update ch"=FALSE, "peak max"=-2147483648.0, "peak min"=2147483648.0, "Weighting Curve"={"Name"="", "Curve"=[], "X data"=1, "Y data"=1, "Z data"=1, "X axis"=0, "Y axis"=1, "Z axis"=1, "X unit"="Hz", "Y unit"="", "Z unit"="deg.", "X dB ref"=1.0, "Y dB ref"=1.0, "Z dB ref"=1.0, "single val"=FALSE, "protected"=FALSE, "display X"=TRUE, "display Y"=TRUE, "display Z"=TRUE, "Test Info"="", "Step No."=0, "Plot Settings"={"Color"=0, "Interpolation"=0, "Point Style"=0, "Line Style"=0, "Point Color"=0, "Line Width"=0, "Bar Plot Style"=0, "Fill To"=0}, "AutoProtect"=FALSE}}] -> w305
            tunnel: w303 -> [w306 _]
            frame False {
            }
            frame True {
            }
          }
        }
        frame 1 {
          n229 = Or(x=w315, y=w314) -> (x .or. y?=w312:bool)
          n230 = case shown="True" w312 {
            tunnel: w310 -> [w317 w325]
            tunnel: [w317 w324] -> w311
            tunnel: w309 -> [w316 w321]
            tunnel: [w316 w319] -> w308
            frame False {
            }
            frame True {
              w322 = FALSE ("Cancel")
              n231 = Bundle By Name(cluster=w325, "halt acq"=TRUE, "acquire"=FALSE) -> (w324:T11)
              n232 = local write "Continue"(w322) -> ()
              n233 = local write "Start"(w322) -> ()
              n234 = Bundle By Name(cluster=w321, "Start"=FALSE) -> (w319:T12)
              n235 = property on="Continue" class="Bool (strict)"("Visible"=w322) -> ()  [unwired: 2 in, 2 out]
            }
          }
        }
        frame 2 {
          n236 = case shown="True" w329 {
            tunnel: w328 -> [w333 w341]
            tunnel: [w333 w340] -> w330
            tunnel: w327 -> [w332 w336]
            tunnel: [w332 w335] -> w326
            frame False {
            }
            frame True {
              w338 = FALSE ("Cancel")
              n237 = local write "Continue"(w338) -> ()
              n238 = local write "Cancel"(w338) -> ()
              n239 = local write "Start"(w338) -> ()
              n240 = property on="Continue" class="Bool (strict)"("Visible"=w338) -> ()  [unwired: 2 in, 2 out]
              n241 = Bundle By Name(cluster=w341, "halt acq"=TRUE, "acquire"=FALSE) -> (w340:T11)
              n242 = Bundle By Name(cluster=w336, "Start"=FALSE) -> (w335:T12)
            }
          }
        }
        frame 3 {
          n243 = Unbundle By Name(w352) -> ("acquire"=w350:bool, "n avgd"=w348:i32, "avg. complete"=w347:i32)
          n244 = Equal To 0?(x=w353) -> (x = 0?=w351:bool)
          n245 = Compound Arithmetic op=AND(w343, w351, w350) -> (w349:bool)
          n246 = case shown="True" w349 {
            tunnel: w352 -> [w356 w364]
            tunnel: [w356 w363] -> w354
            tunnel: w348 -> [_ w362]
            tunnel: w347 -> [_ w361]
            tunnel: w346 -> [_ w360]
            tunnel: w345 -> [w355 w358]
            tunnel: [w355 w357] -> w344
            frame False {
            }
            frame True {
              n247 = Greater Or Equal?(x=w362, y=w361) -> (x >= y?=w359:bool)
              n248 = case shown="True" w359 {
                tunnel: w364 -> [w366 w374]
                tunnel: [w366 w373] -> w363
                tunnel: w360 -> [_ w370]
                tunnel: w358 -> [w365 w368]
                tunnel: [w365 w368] -> w357
                frame False {
                }
                frame True {
                  w371 = FALSE ("Cancel")
                  n249 = case shown="False" w370 {
                    frame False {
                      n250 = local write "OK"(TRUE ("OK")) -> ()
                    }
                    frame True {
                    }
                  }
                  n251 = local write "Continue"(w371) -> ()
                  n252 = local write "Start"(w371) -> ()
                  n253 = property on="Continue" class="Bool (strict)"("Visible"=w371) -> ()  [unwired: 2 in, 2 out]
                  n254 = Bundle By Name(cluster=w374, "n avgd"=0, "halt acq"=TRUE, "acquire"=FALSE) -> (w373:T11)
                }
              }
            }
          }
        }
        frame 4 {
          n255 = Unbundle By Name(w382) -> ("Signal Path"=w383:i32)
          n256 = Not Equal?(x=w383, y=w377) -> (x != y?=w379:bool)
          n257 = case shown="True" w379 {
            tunnel: w381 -> [w384 w385]
            tunnel: [w384 w386] -> w380
            tunnel: w377 -> [_ _]
            frame False {
            }
            frame True {
              n258 = stacked-sequence {
                tunnel: [_ w443 _] -> w386
                tunnel: w385 -> [_ w404 _]
                frame #0 {
                  n259 = local read "Audio Driver"() -> (w387:u16)
                  n260 = case shown="2" w387 {
                    frame 2 {
                      n261 = local read "ASIO_Inited"() -> (w390:bool)
                      n262 = local read "Rcv Idx"() -> (w389:u16)
                      n263 = case shown="True" w390 {
                        frame False {
                        }
                        frame True {
                          n264 = local read "Channel In"() -> (w391:u16)
                          n265 = local read "Asio OCI"() -> (w392:u32)
                          n266 = local write "ASIO_Inited"(FALSE ("ASIO_Inited")) -> ()
                          n267 = call "CRYASIO Close Cur Channel & Dev.vi"("Limit"=w392, "isInput?"=TRUE, "Channel Out"=w391) -> ()  [unwired: 9 in]
                        }
                      }
                      n268 = local read "isMain"() -> (w388:bool)
                      n269 = call "CRYClear Main Receiver Array.vi"("isMain"=w388, "Rcv Idx"=w389) -> ()  [unwired: 10 in]
                    }
                    frame 0, Default {
                      w395 = u32 0 ("nSampleFreq")
                      n270 = local read "Device In"() -> (w398:u32)
                      n271 = local read "taskID"() -> (w396:u32)
                      n272 = dll-call lib="D:/A_CRYSoundLab_Work/CRY6181/CRYSound.dll" fn="GVContinueRecord"("DeviceID"=w398, "nSampleFreq"=w395, "nChannels"=w395, "BitDepth"=w395, "TimeRate"=w395, "mode"=w395, "nBufferUse"=w395, "RealTime"=w395, "timeOut"=w395, "RecData"=i32[] [], "RecDataLen"=w395, "OverHead"=w395, "StartFlag"=w395, "PauseFlag"=w395, "ChangeFlag"=w395, "taskID"=w396) -> ()  [unwired: 9 in, 13 out]
                    }
                  }
                }
                frame #1 {
                  w412 = 4194303.0  # 2^31 - 1
                  (unwired) 2147483647.0  # 2^31 - 1
                  n273 = local read "Manual"() -> (w425:bool)
                  n274 = property on="Signal Path" class="Ring (strict)"() -> ("RingText.Text"=w408:string)  [unwired: 2 in, 2 out]
                  n275 = local read "Hardware in"() -> (w410:string)
                  n276 = local read "Calibration in"() -> (w409:string)
                  n277 = local write "y(n-1)"(0.0) -> ()
                  n278 = local write "Remain Data"(i32[] [] ("Remain Data")) -> ()
                  n279 = case shown="False" w425 {
                    tunnel: [w454 1.0 ("y")] -> w430
                    tunnel: [w452 1.0 ("Y dB ref")] -> w429
                    frame False {
                      n280 = property on="Signal Path" class="Ring (strict)"() -> ("RingText.Text"=w464:string)  [unwired: 2 in, 2 out]
                      n281 = global read "CRYCal Global.vi" "Calibrate"() -> (w457:bool)
                      n282 = global read "CRYCal Global.vi" "Sens In"() -> (w456:dbl)
                      n283 = call "CRYGet Current Calibration Info.vi"("Is Input?"=TRUE, "Signal Type Name"=w464) -> ("Calibration All Cluster"=w465:T6)  [unwired: 9 out]
                      n284 = Unbundle By Name(w465) -> ("Sens Curve.Curve"=w461:cluster{"x":dbl, "y":dbl, "z":dbl}[], "Sens Curve.Y unit"=w459:string, "Sens Curve.Y dB ref"=w453:dbl, "Corr Curve"=→"Corr Curve":T1)
                      n285 = Index Array(array=w461) -> (element=w462:cluster{"x":dbl, "y":dbl, "z":dbl})  [unwired: 1 in]
                      n286 = Match Pattern(string=w459, regular expression="/" ("search char (-)")) -> (after substring=w458:string)  [unwired: 4 out]
                      n287 = Unbundle By Name(w462) -> ("y"=w455:dbl)
                      n288 = case shown="False" w457 {
                        tunnel: [w467 w469] -> w454
                        tunnel: w456 -> [_ w469]
                        tunnel: w455 -> [w467 _]
                        tunnel: [w466 1.0 ("Sens In")] -> w452
                        tunnel: w453 -> [w466 _]
                        frame False {
                        }
                        frame True {
                        }
                      }
                      n289 = local write "dB ref."(w452) -> ()
                      n290 = local write "unit"(w458) -> ()
                    }
                    frame True {
                      n291 = local write "unit"("V" ("unit")) -> ()
                    }
                  }
                  n292 = call "CRYGet Hardware Info From Signal Type.vi"("Calibration In"=w409, "Hardware In"=w410, "Signal Type"=w408, "In/Out?"=TRUE) -> ("Channel Info Out"=w407:T9)  [unwired: 5 in, 2 out]
                  n293 = call "CRYUnit Prefix to Multiplier.vi"() -> ("multiplier"=w436:dbl)  [unwired: 1 in, 4 out]
                  n294 = Unbundle By Name(w407) -> ("Device Name"=w403:string, "Audio Driver"=w402:u16, "ID"=w444:i32, "Sampling Rate (Hz)"=w416:u32, "Bit Depth"=w417:u32, "Hardware Ch ID"=w400:u8, "Vmax (V)"=w406:dbl)
                  n295 = Divide(x=w406, y=w430) -> (x/y=w415:dbl)
                  n296 = Square Root(x=2.0) -> (sqrt(x)=w434:dbl)
                  n297 = case shown="16" w417 {
                    tunnel: [w473 w474 w475 w476] -> w414
                    frame 32, Default {
                      w473 = 2147483647.0  # 2^31 - 1
                    }
                    frame 8 {
                      w474 = 255.0  # 2^8 - 1
                    }
                    frame 16 {
                      w475 = 32767.0  # 2^15 - 1
                    }
                    frame 24 {
                      w476 = 8388607.0  # 2^23 - 1
                    }
                  }
                  n298 = Divide(x=w415, y=w434) -> (x/y=w433:dbl)
                  n299 = Multiply(x=w429, y=w436) -> (x*y=w427:dbl)
                  n300 = Divide(x=w433, y=w427) -> (x/y=w440:dbl)
                  n301 = Logarithm Base 10(1:w440) -> (0:w441:dbl)
                  n302 = Multiply(x=w441, y=20.0) -> (x*y=w426:dbl)
                  n303 = local write "Device Name"(w403) -> ()
                  n304 = local write "Audio Driver"(w402) -> ()
                  n305 = local write "Sampling rate"(w416) -> ()
                  n306 = local write "VMax In"(w406) -> ()
                  n307 = local write "Device In"(w444) -> ()
                  n308 = local write "Channel In"(w400) -> ()
                  n309 = local write "Bits"(w417) -> ()
                  n310 = Add(x=3.0 ("y"), y=w426) -> (x+y=w431:dbl)
                  n311 = Add(x=-90.0, y=w431) -> (x+y=w432:dbl)
                  n312 = Negate(x=w414) -> (-x=w422:dbl)
                  n313 = To Double Precision Float(number=w416) -> (double precision float=w421:dbl)
                  n314 = To Long Integer(number=w417) -> (32bit integer=w420:i32)
                  n315 = property on="dB" class="Slide (strict)"("标尺.范围:最小值"=w432, "标尺.范围:最大值"=w431) -> ()  [unwired: 2 in, 2 out]
                  n316 = property on="Lower limit" class="Slide (strict)"("Scale.Minimum"=w432, "Scale.Maximum"=w431) -> ()  [unwired: 2 in, 2 out]
                  n317 = Bundle(w421, "32bit integer"=2, w420) -> (w418:cluster{dbl, "32bit integer":i32, i32})  [unwired: 1 in]
                  n318 = call "CRYGet Initialized WFM Array.vi"("Sound Format"=w418, "Time(s)"=0.05) -> ("initialized array"=w413:i32[])  [unwired: 8 in, 5 out]
                  n319 = local write "initialized array"(w413) -> ()
                  n320 = local write "Sens"(w430) -> ()
                  n321 = case shown="2" w402 {
                    tunnel: w400 -> [_ w448]
                    frame 0, Default {
                      n322 = local read "Rcv Idx"() -> (w446:u16)
                      n323 = local write "Channels"(u8 2 ("Channels")) -> ()
                      n324 = call "CRYUpdate Receiver Index.vi"("Chn Idx"=-1, "Receiver_Index"=w446) -> ()  [unwired: 9 in]
                    }
                    frame 2 {
                      n325 = local read "Rcv Idx"() -> (w449:u16)
                      n326 = local write "Channels"(u8 1 ("Channels")) -> ()
                      n327 = call "CRYUpdate Receiver Index.vi"("Chn Idx"=w448, "Receiver_Index"=w449) -> ()  [unwired: 9 in]
                    }
                  }
                  n328 = Divide(x=w415, y=w412) -> (x/y=w428:dbl)
                  n329 = Bundle By Name(cluster=w404, "n avgd"=0, "cal factor1"=w428, "cal factor2"=w427, "cal factor3"=w426, "avg. hold"=0.0, "rms max"=w422, "rms min"=w414, "peak max"=w422, "peak min"=w414, "update ch"=TRUE ("update")) -> (w443:T11)
                }
                frame #2 {
                  n330 = local read "ASIO_Inited"() -> (w477:bool)
                  n331 = local read "Audio Driver"() -> (w478:u16)
                  n332 = case shown="2" w478 {
                    tunnel: w477 -> [w479 _]
                    frame 2 {
                      n333 = case shown="False" w479 {
                        frame False {
                          n334 = local read "Device Name"() -> (w488:string)
                          n335 = local read "Sampling rate"() -> (w486:u32)
                          n336 = local read "Bits"() -> (w485:u32)
                          n337 = local read "Channel In"() -> (w487:u16)
                          n338 = local read "Rcv Idx"() -> (w482:u16)
                          n339 = call "CRYSet Main Receiver Array.vi"("Rcv Idx"=w482) -> ("Is Main?"=w481:bool)  [unwired: 10 in]
                          n340 = call "CRYASIO In & Init & Start.vi"("Bit Depth"=w485, "Sampling Rate"=w486, "Channel Index"=w487, "Device Name"=w488) -> ("bResult"=w483:bool, "ASIO Opend Channel Index"=→"Asio OCI":u32)  [unwired: 6 in]
                          n341 = local write "ASIO_Inited"(w483) -> ()
                          n342 = local write "Buf Cnt"(-1 ("Buf Cnt")) -> ()
                          n343 = local write "isMain"(w481) -> ()
                        }
                        frame True {
                        }
                      }
                    }
                    frame 0, Default {
                      n344 = local write "start_flg"(u8 1 ("start_flg")) -> ()
                    }
                  }
                }
              }
            }
          }
        }
        frame 5 {
          n345 = Unbundle By Name(w494) -> ("Continue"=w495:bool)
          n346 = Not Equal?(x=w495, y=w491) -> ()  [unwired: 1 out]
        }
        frame 6 {
          n347 = Unbundle By Name(w501) -> ("Mode"=w500:i32)
          n348 = Not Equal?(x=w500, y=w498) -> (x != y?=w499:bool)
          n349 = case shown="True" w499 {
            tunnel: w498 -> [_ w504]
            frame False {
            }
            frame True {
              n350 = case shown="0, Default" w504 {
                tunnel: [u8 2 ("Display Format:Precision") u8 0 ("Display Format:Precision")] -> w503
                frame 0, Default {
                  n351 = property on="Level" class="Slide (strict)"("Value"=u8 0 ("Display Format:Precision")) -> ()  [unwired: 2 in, 2 out]
                }
                frame 1, 2 {
                }
              }
              n352 = property on="Level" class="Slide (strict)"("Disabled"=w503) -> ()  [unwired: 2 in, 2 out]
            }
          }
        }
        frame 7 {
          n353 = Unbundle By Name(w512) -> ("Level"=w513:i32)
          n354 = Not Equal?(x=w513, y=w511) -> ()  [unwired: 1 out]
        }
        frame 8 {
          n355 = Unbundle By Name(w522) -> ("Lin/Exp"=w523:i32)
          n356 = Not Equal?(x=w523, y=w519) -> (x != y?=w520:bool)
          n357 = case shown="True" w520 {
            tunnel: w519 -> [_ w536]
            tunnel: w518 -> [w524 w529]
            tunnel: [w524 w535] -> w517
            tunnel: w516 -> [_ w531]
            tunnel: w514 -> [_ w527]
            frame False {
            }
            frame True {
              n358 = case shown="0, Default" w536 {
                tunnel: [w539 w548] -> w526
                tunnel: w531 -> [_ w557]
                tunnel: w529 -> [w543 w555]
                tunnel: [w544 w554] -> w528
                tunnel: w527 -> [w542 _]
                frame 0, Default {
                  n359 = Divide(x=w542, y=0.05) -> (x/y=w545:dbl)
                  n360 = Bundle By Name(cluster=w543, "avg. complete"=w545) -> (w544:T11)
                  n361 = call "CRYGet Error Message.vi"("Error No"=0, "Kind"="Multimeter Sub") -> ("Unicode Message Sub"=w539:string[])  [unwired: 4 in, 5 out]
                  n362 = local write "Elapsed Time"(0.0 ("Elapsed Time")) -> ()
                }
                frame 1 {
                  n363 = case shown="0, Default" w557 {
                    tunnel: [u8 2 ("Disabled") u8 2 ("Disabled") u8 0 ("Disabled")] -> w556
                    tunnel: [0.25 ("Avg.Time(sec)") 2.0 ("Avg.Time(sec)") w563] -> w553
                    frame 0, Default {
                    }
                    frame 1 {
                    }
                    frame 2 {
                      n364 = local read "User Avg.Time(sec)"() -> (w563:dbl)
                    }
                  }
                  n365 = property on="Continue" class="Bool (strict)"("Visible"=FALSE) -> ()  [unwired: 2 in, 2 out]
                  n366 = Divide(x=w553, y=0.05) -> (x/y=w551:dbl)
                  n367 = property on="Avg.Time(sec)" class="DigNum (strict)"("Disabled"=w556) -> ()  [unwired: 2 in, 2 out]
                  n368 = property on="Avg.Time(sec)" class="DigNum (strict)"("Value"=w553) -> ()  [unwired: 2 in, 2 out]
                  n369 = Bundle By Name(cluster=w555, "avg. complete"=w551) -> (w554:T11)
                  n370 = call "CRYGet Error Message.vi"("Error No"=1, "Kind"="Multimeter Sub") -> ("Unicode Message Sub"=w548:string[])  [unwired: 4 in, 5 out]
                }
              }
              n371 = Equal To 0?(x=w536) -> (x = 0?=w533:bool)
              n372 = property on="Time(sec)" class="DigNum (strict)"("Visible"=w533) -> ()  [unwired: 2 in, 2 out]
              n373 = property on="Elapsed Time" class="DigNum (strict)"("Visible"=w533) -> ()  [unwired: 2 in, 2 out]
              n374 = Not(x=w533) -> (.not. x?=w532:bool)
              n375 = property on="Time Weighting" class="Ring (strict)"("Visible"=w532) -> ()  [unwired: 2 in, 2 out]
              n376 = property on="Avg.Time(sec)" class="DigNum (strict)"("Visible"=w532) -> ()  [unwired: 2 in, 2 out]
              n377 = Bundle By Name(cluster=w528, "n avgd"=0 ("avg. complete"), "update"=TRUE) -> (w535:T11)
              n378 = for {
                tunnel: w526 -> [w538] mode=indexing
                tunnel: [w537] -> w525 mode=indexing
                n379 = call "CRYConvert Unicode to ASCII.vi"("Unicode"=w538) -> ("ASCII"=w537:string)  [unwired: 4 in]
              }
              n380 = property on="Start" class="Bool (strict)"("Strings [4]"=w525) -> ()  [unwired: 2 in, 2 out]
            }
          }
        }
        frame 9 {
          n381 = Unbundle By Name(w571) -> ("Weighting"=w572:i32)
          n382 = Not Equal?(x=w572, y=w565) -> (x != y?=w568:bool)
          n383 = case shown="True" w568 {
            tunnel: w565 -> [_ w578]
            tunnel: w567 -> [w573 w575]
            tunnel: [w573 w580] -> w566
            frame False {
            }
            frame True {
              n384 = property on="Weighting" class="Ring (strict)"() -> ("Strings []"=w576:string[])  [unwired: 2 in, 2 out]
              n385 = Index Array(array=w576, index=w578) -> (element=w577:string)
              n386 = call "CRYGet Weighting Value.vi"("Weighting Name"=w577) -> ("Weighting Curve"=w574:T1)  [unwired: 10 in]
              n387 = Bundle By Name(cluster=w575, "Weighting Curve"=w574, "update"=TRUE) -> (w580:T11)
            }
          }
        }
        frame 10 {
          n388 = Unbundle By Name(w585) -> ("Apply Correction"=w586:bool)
          n389 = Not Equal?(x=w586, y=w584) -> ()  [unwired: 1 out]
        }
        frame 11 {
          n390 = Unbundle By Name(w592) -> ("Limits On"=w593:bool)
          n391 = Not Equal?(x=w593, y=w590) -> (x != y?=w591:bool)
          n392 = case shown="True" w591 {
            tunnel: w590 -> [_ w594]
            frame False {
            }
            frame True {
              n393 = global write "CRYLimit edit global.vi" "Limits On"(w594) -> ()
              n394 = property on="Upper Str" class="Bool (strict)"("Visible"=w594) -> ()  [unwired: 2 in, 2 out]
              n395 = property on="Lower Str" class="Bool (strict)"("Visible"=w594) -> ()  [unwired: 2 in, 2 out]
              n396 = property on="Verdict" class="Bool (strict)"("可见"=w594) -> ()  [unwired: 2 in, 2 out]
              n397 = property on="Lower limit" class="Slide (strict)"("Visible"=w594) -> ()  [unwired: 2 in, 2 out]
            }
          }
        }
        frame 12 {
          n398 = Unbundle By Name(w600) -> ("Time Weighting"=w601:i32)
          n399 = Not Equal?(x=w601, y=w595) -> (x != y?=w596:bool)
          n400 = case shown="True" w596 {
            tunnel: w595 -> [_ w602]
            frame False {
            }
            frame True {
              n401 = case shown="2" w602 {
                tunnel: [u8 2 ("Disabled") u8 2 ("Disabled") u8 0 ("Disabled")] -> w604
                tunnel: [0.25 ("Avg.Time(sec)") 2.0 ("Avg.Time(sec)") w615] -> w603
                frame 0, Default {
                }
                frame 1 {
                }
                frame 2 {
                  n402 = local read "User Avg.Time(sec)"() -> (w615:dbl)
                }
              }
              n403 = disable-structure shown="禁用" {
                disable-tunnel: w603 -> [w605 _]
                frame Disabled {
                  n404 = Less?(x=w605, y=1.0) -> (x < y?=w607:bool)
                  n405 = case shown="True" w607 {
                    tunnel: [u8 2 ("Display Format:Precision") u8 0 ("Display Format:Precision")] -> w608
                    frame False {
                    }
                    frame True {
                    }
                  }
                  n406 = property on="Avg.Time(sec)" class="DigNum (strict)"("Precision"=w608) -> ()  [unwired: 2 in, 2 out]
                }
                frame Enabled {
                }
              }
              n407 = property on="Avg.Time(sec)" class="DigNum (strict)"("Disabled"=w604) -> ()  [unwired: 2 in, 2 out]
              n408 = local write "Avg.Time(sec)"(w603) -> ()
            }
          }
        }
        frame 13 {
          n409 = Unbundle By Name(w624) -> ("Time(sec)"=w625:dbl)
          n410 = Not Equal?(x=w625, y=w622) -> (x != y?=w623:bool)
          n411 = case shown="True" w623 {
            tunnel: w622 -> [_ w627]
            tunnel: w619 -> [w626 w637]
            tunnel: [w626 w636] -> w618
            tunnel: w617 -> [_ _]
            frame False {
            }
            frame True {
              w631 = 10.0 ("y")
              w632 = 0.05 ("y")
              n412 = Greater?(x=w632, y=w627) -> (0:w633:bool)
              n413 = Select(t=w632, s=w633, f=w627) -> (s? t:f=w629:dbl)
              n414 = Divide(x=w627, y=0.05) -> (x/y=w638:dbl)
              n415 = Less?(x=w631, y=w629) -> (x < y?=w630:bool)
              n416 = To Long Integer(number=w638) -> (32bit integer=w634:i32)
              n417 = Select(t=w631, s=w630, f=w629) -> (s? t:f=w628:dbl)
              n418 = local write "Time(sec)"(w628) -> ()
              n419 = Bundle By Name(cluster=w637, "avg. complete"=w634, "update"=TRUE) -> (w636:T11)
            }
          }
        }
        frame 14 {
          n420 = Unbundle By Name(w651) -> ("Avg.Time(sec)"=w650:dbl)
          n421 = Not Equal?(x=w650, y=w645) -> (x != y?=w640:bool)
          n422 = Equal?(x=2 ("y"), y=w649) -> (x = y?=w641:bool)
          n423 = case shown="True" w640 {
            tunnel: w645 -> [_ w655]
            tunnel: w644 -> [w652 w658]
            tunnel: [w652 w660] -> w643
            tunnel: w642 -> [_ w659]
            tunnel: w640 -> [_ _]
            tunnel: w641 -> [_ w653]
            frame False {
            }
            frame True {
              n424 = Divide(x=w655, y=0.05 ("x")) -> (x/y=w657:dbl)
              n425 = To Long Integer(number=w657) -> (32bit integer=w654:i32)
              n426 = case shown="True" w653 {
                tunnel: w655 -> [_ w661]
                frame False {
                }
                frame True {
                  n427 = local write "User Avg.Time(sec)"(w661) -> ()
                }
              }
              n428 = case shown="1" w659 {
                tunnel: w658 -> [w662 w666]
                tunnel: [w662 w665] -> w660
                tunnel: w654 -> [_ w663]
                frame 0, Default {
                }
                frame 1 {
                  n429 = Bundle By Name(cluster=w666, "avg. complete"=w663, "update"=TRUE) -> (w665:T11)
                }
              }
            }
          }
        }
        frame 15 {
          n430 = Unbundle By Name(w679) -> ("Start"=w668:bool)
          n431 = Not Equal?(x=w668, y=w671) -> (x != y?=w674:bool)
          n432 = And(x=w674, y=w671) -> (x .and. y?=w680:bool)
          n433 = Compound Arithmetic op=OR(w680, w670) -> (w678:bool)
          n434 = case shown="True" w678 {
            tunnel: w677 -> [w687 w742]
            tunnel: [w686 w735] -> w676
            tunnel: w675 -> [w685 w734]
            tunnel: w673 -> [w689 w740]
            tunnel: [w688 w739] -> w672
            tunnel: w671 -> [w683 _]
            tunnel: w670 -> [_ w745]
            tunnel: w669 -> [_ w726]
            tunnel: w668 -> [w684 _]
            tunnel: w667 -> [_ w725]
            frame False {
              n435 = Not Equal?(x=w684, y=w683) -> (x != y?=w682:bool)
              n436 = case shown="True" w682 {
                tunnel: w689 -> [w691 w696]
                tunnel: [w691 w694] -> w688
                tunnel: w687 -> [w690 w702]
                tunnel: [w690 w705] -> w686
                tunnel: w685 -> [_ w704]
                frame False {
                }
                frame True {
                  w693 = FALSE ("Conflag")
                  n437 = Unbundle By Name(w702) -> ("n avgd"=w697:i32, "avg. complete"=w701:i32)
                  n438 = local read "Audio Driver"() -> (w692:u16)
                  n439 = case shown="2" w692 {
                    frame 0, Default {
                      w708 = 0.0 ("nSampleFreq")
                      w710 = u8 0 ("nSampleFreq")
                      w709 = u32 0 ("nSampleFreq")
                      n440 = local read "Device In"() -> (w713:u32)
                      n441 = local read "taskID"() -> (w711:u32)
                      n442 = dll-call lib="D:/A_CRYSoundLab_Work/CRY6181/CRYSound.dll" fn="GVContinueRecord"("DeviceID"=w713, "nSampleFreq"=w709, "nChannels"=w709, "BitDepth"=w709, "TimeRate"=w708, "mode"=w709, "nBufferUse"=w709, "RealTime"=w709, "timeOut"=w708, "RecData"=i32[] [], "RecDataLen"=w709, "OverHead"=w710, "StartFlag"=w710, "PauseFlag"=w710, "ChangeFlag"=w710, "taskID"=w711) -> ()  [unwired: 14 in, 8 out]
                    }
                    frame 2 {
                    }
                  }
                  n443 = Equal To 0?(x=w704) -> (x = 0?=w703:bool)
                  n444 = Not Equal To 0?(x=w697) -> (x != 0?=w698:bool)
                  n445 = Less?(x=w697, y=w701) -> (x < y?=w699:bool)
                  n446 = Compound Arithmetic op=AND(w703, w698, w699) -> (w700:bool)
                  n447 = property on="Continue" class="Bool (strict)"("Visible"=w700) -> ()  [unwired: 2 in, 2 out]
                  n448 = case shown="True" w700 {
                    frame False {
                    }
                    frame True {
                      n449 = call "CRYGet Error Message.vi"("Error No"=2, "Kind"="Multimeter Sub") -> ("Unicode Message Sub"=w715:string[])  [unwired: 4 in, 5 out]
                      n450 = for {
                        tunnel: w715 -> [w719] mode=indexing
                        tunnel: [w718] -> w714 mode=indexing
                        n451 = call "CRYConvert Unicode to ASCII.vi"("Unicode"=w719) -> ("ASCII"=w718:string)  [unwired: 4 in]
                      }
                      n452 = property on="Start" class="Bool (strict)"("Strings [4]"=w714) -> ()  [unwired: 2 in, 2 out]
                    }
                  }
                  n453 = local write "Continue"(w693) -> ()
                  n454 = local write "AveString"(w693) -> ()
                  n455 = local write "Start"(w693) -> ()
                  n456 = Bundle By Name(cluster=w696, "Start"=FALSE) -> (w694:T12)
                  n457 = Bundle By Name(cluster=w702, "acquire"=FALSE, "halt acq"=TRUE) -> (w705:T11)
                }
              }
            }
            frame True {
              w746 = TRUE ("Conflag")
              w744 = FALSE ("Visible")
              # "???"
              n458 = local write "Continue"(w744) -> ()
              n459 = property on="Continue" class="Bool (strict)"("Visible"=w744) -> ()  [unwired: 2 in, 2 out]
              n460 = local write "AveString"(w746) -> ()
              n461 = local write "y(n-1)"(0.0) -> ()
              n462 = local write "Start"(w746) -> ()
              n463 = local write "Remain Data"(i32[] [] ("Remain Data")) -> ()
              n464 = local read "Bits"() -> (w737:u32)
              n465 = case shown="0, Default" w734 {
                tunnel: w726 -> [w752 _]
                tunnel: w725 -> [_ w756]
                tunnel: [w752 w756] -> w731
                tunnel: [w749 w753] -> w724
                frame 0, Default {
                  n466 = call "CRYGet Error Message.vi"("Error No"=0, "Kind"="Multimeter Sub") -> ("Unicode Message Sub"=w749:string[])  [unwired: 4 in, 5 out]
                }
                frame 1 {
                  n467 = call "CRYGet Error Message.vi"("Error No"=1, "Kind"="Multimeter Sub") -> ("Unicode Message Sub"=w753:string[])  [unwired: 4 in, 5 out]
                }
              }
              n468 = Divide(x=w731, y=0.05) -> (x/y=w733:dbl)
              n469 = To Long Integer(number=w733) -> (32bit integer=w732:i32)
              n470 = Bundle By Name(cluster=w742, "avg. complete"=w732) -> (w741:T11)
              n471 = case shown="16" w737 {
                tunnel: [w757 w758 w759 w760] -> w727
                frame 8 {
                  w757 = 255.0  # 2^8 - 1
                }
                frame 16 {
                  w758 = 32767.0  # 2^15 - 1
                }
                frame 24 {
                  w759 = 524287.0  # 2^19 - 1
                }
                frame 32, Default {
                  w760 = 4194303.0  # 2^22 - 1
                }
              }
              n472 = Bundle By Name(cluster=w740, "Start"=TRUE) -> (w739:T12)
              n473 = case shown="True" w745 {
                tunnel: [w764 w768] -> w736
                tunnel: w741 -> [w761 w767]
                frame False {
                  n474 = Bundle By Name(cluster=w761, "acquire"=TRUE ("Bundle Element"), "halt acq"=FALSE, "n avgd"=0 ("Bundle Element")) -> (w764:T11)
                }
                frame True {
                  n475 = Unbundle By Name(w767) -> ("avg. complete"=w766:i32, "n avgd"=w772:i32)
                  n476 = Bundle By Name(cluster=w767, "acquire"=TRUE ("Bundle Element"), "halt acq"=FALSE) -> (w770:T11)
                  n477 = Less Or Equal?(x=w766, y=w772) -> (x <= y?=w771:bool)
                  n478 = case shown="True" w771 {
                    tunnel: w770 -> [w774 w776]
                    tunnel: [w774 w775] -> w768
                    frame False {
                    }
                    frame True {
                      n479 = Bundle By Name(cluster=w776, "n avgd"=0) -> (w775:T11)
                    }
                  }
                }
              }
              n480 = Negate(x=w727) -> (-x=w728:dbl)
              n481 = Bundle By Name(cluster=w736, "avg. hold"=0.0, "rms max"=w728, "rms min"=w727, "peak max"=w728, "peak min"=w727, "update"=TRUE) -> (w735:T11)
              n482 = for {
                tunnel: w724 -> [w748] mode=indexing
                tunnel: [w747] -> w723 mode=indexing
                n483 = call "CRYConvert Unicode to ASCII.vi"("Unicode"=w748) -> ("ASCII"=w747:string)  [unwired: 4 in]
              }
              n484 = local write "start_flg"(u8 1 ("start_flg")) -> ()
              n485 = property on="Start" class="Bool (strict)"("Strings [4]"=w723) -> ()  [unwired: 2 in, 2 out]
            }
          }
        }
        frame Default {
          n486 = Unbundle By Name(w800) -> ("Time(sec)"=w801:dbl, "Lin/Exp"=w796:i32, "Avg.Time(sec)"=w794:dbl)
          n487 = Wait (ms)(milliseconds to wait=u32 20) -> ()  [unwired: 1 out]
          n488 = Not Equal?(x=w801, y=w799) -> (x != y?=w798:bool)
          n489 = Not Equal?(x=w796, y=w788) -> (x != y?=w795:bool)
          n490 = Not Equal?(x=w794, y=w793) -> (x != y?=w792:bool)
          n491 = Compound Arithmetic op=OR(w789, w798, w795, w792) -> (w797:bool)
          n492 = case shown="True" w797 {
            tunnel: w788 -> [_ w810]
            tunnel: w791 -> [w804 w809]
            tunnel: [w804 w808] -> w790
            frame False {
            }
            frame True {
              n493 = Unbundle By Name(w809) -> ("avg. complete"=w805:i32)
              n494 = case shown="1" w810 {
                tunnel: [w813 w817] -> w807
                tunnel: w805 -> [w812 w814]
                frame 0, Default {
                  # "uniform weighting"
                  n495 = Reciprocal(x=w812) -> (1/x=w811:dbl)
                  n496 = Initialize Array(w811, w812) -> (w813:dbl[])
                }
                frame 1 {
                  # "exponential weighting"
                  n497 = Greater?(x=w814, y=1) -> (0:w815:bool)
                  n498 = case shown="True" w815 {
                    tunnel: [dbl[] [1.0] w827] -> w817
                    tunnel: w814 -> [_ w826]
                    frame False {
                    }
                    frame True {
                      w821 = -3.5  # last pt taus
                      n499 = Decrement(x=w826) -> (x-1=w820:i32)
                      n500 = Divide(x=w821, y=w820) -> (x/y=w819:dbl)
                      n501 = for {
                        N: w826 -> [_]
                        tunnel: [w828] -> w824 mode=indexing
                        tunnel: w819 -> [w830]
                        i -> [w829]
                        n502 = Multiply(x=w829, y=w830) -> (x*y=w828:dbl)
                      }
                      n503 = Exponential(1:w824) -> (0:w822:dbl[])
                      n504 = Add Array Elements(numeric array=w822) -> (sum=w825:dbl)
                      n505 = Divide(x=w822, y=w825) -> (x/y=w823:dbl[])
                      n506 = Reverse 1D Array(array=w823) -> (reversed array=w827:dbl[])
                    }
                  }
                }
              }
              n507 = Bundle By Name(cluster=w809, "Avg.weighting"=w807, "update"=TRUE) -> (w808:T11)
            }
          }
          n508 = Unbundle("Lower limit") -> (w779:dbl, w778:dbl)
          n509 = Max & Min(x=w779, y=w778) -> (max(x,y)=w783:dbl, min(x,y)=w784:dbl)
          n510 = Bundle(w783, w784) -> (w781:cluster{dbl, dbl})  [unwired: 1 out]
          n511 = local read "dB"() -> (w785:cluster{dbl, dbl})
          n512 = local write "Lower limit"(w781) -> ()
          n513 = Unbundle(w785) -> (w786:dbl)  [unwired: 1 out]
          n514 = In Range and Coerce(upper limit=w783, x=w786, lower limit=w784) -> (In Range?=→"Verdict":bool)  [unwired: 1 out]
        }
      }
    }
    n515 = Unbundle By Name(w235) -> ("acquire"=w242:bool)
    n516 = case "stop?" shown="True" w242 {
      tunnel: w273 -> [w834 w952]
      tunnel: w274 -> [w835 w954]
      tunnel: w267 -> [w836 w907]
      tunnel: [w836 w905] -> w276
      tunnel: [w835 w953] -> w275
      tunnel: [w834 w951] -> w264
      tunnel: w235 -> [w833 w874]
      tunnel: w243 -> [_ w942]
      tunnel: [w833 w920] -> w244
      frame False {
        n517 = local read "Audio Driver"() -> (w831:u16)
        n518 = case shown="2" w831 {
          frame 2 {
            n519 = local read "Rcv Idx"() -> (w837:u16)
            n520 = call "CRYCheck Main Receiver.vi"("Rcv Idx"=w837) -> ("Is Main?"=w839:bool)  [unwired: 10 in]
            n521 = local read "ASIO_Inited"() -> (w838:bool)
            n522 = local write "isMain"(w839) -> ()
            n523 = And(x=w838, y=w839) -> (x .and. y?=w840:bool)
            n524 = case shown="False" w840 {
              tunnel: w837 -> [_ w842]
              frame False {
                n525 = local write "Buf Cnt"(-1 ("Buf Cnt")) -> ()
              }
              frame True {
                n526 = local read "Asio OCI"() -> (w845:u32)
                n527 = call "CRYASIO Receive Data.vi"("Rcv Idx"=w842, "Limit"=w845, "Data Length"=2048, "Last Remain Buffer"=i32[] []) -> ()  [unwired: 5 in, 3 out]
              }
            }
          }
          frame 0, Default {
          }
        }
        n528 = Wait (ms)(milliseconds to wait=u32 20) -> ()  [unwired: 1 out]
      }
      frame True {
        w918 = u8 0 ("StartFlag")
        w881 = 0.05 ("y")
        w916 = FALSE ("halt acq")
        # "RMS"
        # "Peak"
        n529 = local read "initialized array"() -> (w898:i32[])
        n530 = local read "Audio Driver"() -> (w880:u16)
        n531 = local read "Sampling rate"() -> (w892:u32)
        n532 = local read "Channel In"() -> (w890:u16)
        n533 = local read "Device In"() -> (w947:u32)
        n534 = local read "Channels"() -> (w950:u8)
        n535 = local read "Bits"() -> (w948:u32)
        n536 = Unbundle By Name(w874) -> ("avg. complete"=w876:i32, "n avgd"=w901:i32, "halt acq"=w938:bool, "update ch"=w917:bool)
        n537 = Boolean To (0,1)(Boolean=w917) -> (0, 1=w919:i16)
        n538 = local read "Lin/Exp"() -> (w900:i32)
        n539 = Equal To 0?(x=w880) -> (x = 0?=w888:bool)
        n540 = Not(x=w938) -> (.not. x?=w939:bool)
        n541 = Select(t=0.1 ("x"), s=w888, f=w881) -> (s? t:f=w889:dbl)
        n542 = Multiply(x=w881, y=w876) -> (x*y=w914:dbl)
        n543 = Multiply(x=w892, y=w914) -> (x*y=w913:dbl)
        n544 = Multiply(x=w889, y=w892) -> (x*y=w909:dbl)
        n545 = To Long Integer(number=w909) -> (32bit integer=w908:i32)
        n546 = while {
          tunnel: w942 -> [w1070]
          shift-right: [w1074] -> w941
          shift-left: i32[] [] -> [w1051]
          shift-right: [w1068] -> w940
          shift-left: w918 -> [w1073]
          tunnel: 0.05 ("TimeRate") -> [w1067]
          tunnel: 0.0 ("timeOut") -> [w1066]
          tunnel: w918 -> [w1065]
          tunnel: u8 1 ("StartFlag") -> [w1064]
          tunnel: w947 -> [w1063]
          tunnel: w892 -> [w1062]
          tunnel: w948 -> [w1061]
          tunnel: u32 0 ("mode") -> [w1060]
          tunnel: w950 -> [w1059]
          tunnel: w938 -> [w1058]
          tunnel: [w1057] -> w925
          shift-right: [i16 0] -> _
          shift-left: w919 -> [w1056]
          tunnel: w908 -> [w1053]
          tunnel: w898 -> [w1052]
          tunnel: w880 -> [w1050]
          tunnel: w890 -> [w1049]
          stop <- w1069 continue-if-true
          n547 = case shown="0, Default" w1050 {
            tunnel: [w1080 w1135] -> w1074
            tunnel: w1073 -> [w1083 w1133]
            tunnel: [w1082 w1132] -> w1068
            tunnel: w1067 -> [_ w1131]
            tunnel: w1066 -> [_ w1130]
            tunnel: w1065 -> [_ w1129]
            tunnel: w1064 -> [_ _]
            tunnel: w1063 -> [_ w1123]
            tunnel: w1062 -> [_ w1122]
            tunnel: w1061 -> [_ w1121]
            tunnel: w1060 -> [_ w1120]
            tunnel: w1059 -> [_ w1119]
            tunnel: [w1084 w1118] -> w1057
            tunnel: w1056 -> [_ w1117]
            tunnel: w1053 -> [w1085 w1116]
            tunnel: w1052 -> [_ w1115]
            tunnel: w1051 -> [_ w1113]
            tunnel: w1049 -> [w1077 _]
            frame 2 {
              # "ASIO"
              n548 = local read "Rcv Idx"() -> (w1079:u16)
              n549 = call "CRYCheck Main Receiver.vi"("Rcv Idx"=w1079) -> ("Is Main?"=w1078:bool)  [unwired: 10 in]
              n550 = local read "ASIO_Inited"() -> (w1081:bool)
              n551 = case shown="True" w1081 {
                tunnel: w1085 -> [w1086 w1095]
                tunnel: [0 ("Over Load") w1094] -> w1084
                tunnel: [w1088 w1093] -> w1080
                tunnel: w1079 -> [_ w1092]
                tunnel: w1078 -> [_ w1091]
                tunnel: w1077 -> [_ w1090]
                frame False {
                  n552 = Initialize Array(0 ("element"), w1086) -> (w1088:i32[])
                }
                frame True {
                  n553 = case shown="False" w1091 {
                    tunnel: w1095 -> [w1101 w1109]
                    tunnel: [w1100 w1108] -> w1094
                    tunnel: [w1098 w1107] -> w1093
                    tunnel: w1092 -> [w1096 _]
                    tunnel: w1090 -> [_ w1105]
                    frame True {
                      n554 = local read "Remain Data"() -> (w1102:i32[])
                      n555 = local read "Asio OCI"() -> (w1099:u32)
                      n556 = call "CRYASIO Receive Data.vi"("Rcv Idx"=w1096, "Limit"=w1099, "Data Length"=w1101, "Last Remain Buffer"=w1102) -> ("Over Load"=w1100:i32, "Data Out"=w1098:i32[], "Remain Data"=w1097:i32[])  [unwired: 5 in]
                      n557 = local write "Remain Data"(w1097) -> ()
                    }
                    frame False {
                      n558 = local read "Remain Data"() -> (w1110:i32[])
                      n559 = local read "Buf Cnt"() -> (w1103:i32)
                      n560 = call "CRYASIO Receive Global Data.vi"("buf count"=w1103, "Chn Idx"=w1105, "Data Length"=w1109, "Last Remain Buffer"=w1110) -> ("Over Load"=w1108:i32, "bufCount"=w1104:i32, "Data Out"=w1107:i32[], "Remain Data"=w1106:i32[])  [unwired: 4 in]
                      n561 = local write "Buf Cnt"(w1104) -> ()
                      n562 = local write "Remain Data"(w1106) -> ()
                    }
                  }
                }
              }
              n563 = local write "isMain"(w1078) -> ()
              n564 = Increment(x=w1083) -> (x+1=w1082:u8)
            }
            frame 0, Default {
              n565 = local read "start_flg"() -> (w1112:u8)
              n566 = dll-call lib="D:/A_CRYSoundLab_Work/CRY6181/CRYSound.dll" fn="GVContinueRecord"("DeviceID"=w1123, "nSampleFreq"=w1122, "nChannels"=w1119, "BitDepth"=w1121, "TimeRate"=w1131, "mode"=w1120, "timeOut"=w1130, "RecData"=w1115, "StartFlag"=w1112, "PauseFlag"=w1129, "ChangeFlag"=w1117, "taskID"="taskID") -> ("return type"=w1111:u32, "nBufferUse"=→"nBufferUse":u32, "RealTime"=→"RealTime":u32, "RecData"=w1114:i32[], "RecDataLen"=w1126:u32, "OverHead"=w1118:u8, "taskID"=w1127:u32)  [unwired: 12 in, 7 out]
              "OverHead" <- w1118
              "return type" <- w1111
              n567 = local write "taskID"(w1127) -> ()
              n568 = case shown="0, Default" w1111 {
                frame 0, Default {
                }
                frame 2 {
                  n569 = local write "start_flg"(u8 0 ("start_flg")) -> ()
                  n570 = local write "Start"(FALSE ("Start")) -> ()
                }
              }
              n571 = Equal To 0?(x=w1126) -> (x = 0?=w1134:bool)
              n572 = case shown="False" w1134 {
                tunnel: w1114 -> [w1140 _]
                tunnel: w1113 -> [w1144 w1147]
                tunnel: [w1143 w1147] -> w1135
                tunnel: w1133 -> [w1142 w1146]
                tunnel: [w1141 w1146] -> w1132
                tunnel: w1116 -> [w1139 _]
                frame False {
                  n573 = Array Subset(array=w1140, length=w1139) -> (w1138:i32[])  [unwired: 1 in]
                  n574 = Increment(x=w1142) -> (x+1=w1141:u8)
                  n575 = Build Array (concatenate)(w1144, w1138) -> (w1143:i32[])
                }
                frame True {
                  n576 = Wait (ms)(milliseconds to wait=u32 10) -> ()  [unwired: 1 out]
                }
              }
            }
          }
          n577 = local read "start_flg"() -> (w1048:u8)
          n578 = Equal To 0?(x=w1048) -> (x = 0?=w1047:bool)
          n579 = local read "Cancel"() -> (w1075:bool)
          n580 = local read "OK"() -> (w1076:bool)
          n581 = Not Or(1:w1075, 2:w1076) -> (0:w1071:bool)
          n582 = Less?(x=w1068, y=1 ("buffers")) -> (x < y?=w1072:bool)
          n583 = Compound Arithmetic op=AND(invert w1047, invert w1058, invert w1070, w1072, w1071) -> (w1069:bool)
        }
        n584 = case shown="0" w900 {
          tunnel: w940 -> [w1001 w1006]
          tunnel: [w999 w1005] -> w921
          tunnel: w901 -> [w998 w1004]
          tunnel: w876 -> [w1002 _]
          frame 1, Default {
            n585 = Greater Or Equal?(x=w998, y=w1002) -> (x >= y?=w1003:bool)
            n586 = Add(x=w1001, y=w998) -> (x+y=w1000:i32)
            n587 = Select(t=w1001, s=w1003, f=w1000) -> (s? t:f=w999:i32)
          }
          frame 0 {
            n588 = Add(x=w1006, y=w1004) -> (x+y=w1005:i32)
          }
        }
        n589 = To Long Integer(number=w913) -> ()  [unwired: 1 out]
        n590 = Multiply(x=w921, y=0.05) -> (x*y=w923:dbl)
        n591 = Bundle By Name(cluster=w874, "n avgd"=w921, "acquire"=w939, "halt acq"=w916, "update"=w916, "update ch"=w916) -> (w891:T11)
        n592 = local write "Elapsed Time"(w923) -> ()
        n593 = Subtract(x=w907, y=w876) -> (x-y=w937:i32)
        n594 = Greater Or Equal To 0?(x=w937) -> (x >= 0?=w902:bool)
        n595 = case "buffer full, at least?" shown="True" w902 {
          tunnel: [w1028 w1035] -> w930
          tunnel: w954 -> [w1028 w1036]
          tunnel: w937 -> [_ w1034]
          tunnel: w907 -> [w1027 w1033]
          tunnel: [w1027 w1032] -> w927
          tunnel: w952 -> [w1026 w1030]
          tunnel: [w1026 w1029] -> w931
          frame False {
          }
          frame True {
            n596 = Increment(x=w1034) -> (x+1=w1031:i32)
            n597 = for {
              N: w1031 -> [_]
              shift-right: [w1040] -> w1032
              shift-left: w1033 -> [w1041]
              shift-right: [w1038] -> w1035
              shift-left: w1036 -> [_]
              tunnel: w1030 -> [w1039]
              tunnel: [w1037] -> w1029
              n598 = Dequeue Element(queue=w1039) -> (queue out=w1037:refnum<queue>, error out=w1038:errorcluster)  [unwired: 1 in, 3 out]
              n599 = Decrement(x=w1041) -> (x-1=w1040:i32)
            }
          }
        }
        n600 = local read "Channel In"() -> (w884:u16)
        n601 = Unbundle By Name(w874) -> ("avg. complete"=w868:i32, "cal factor1"=w879:dbl, "cal factor2"=w903:dbl, "cal factor3"=w899:dbl, "rms max"=w862:dbl, "rms min"=w912:dbl, "peak max"=w911:dbl, "peak min"=w861:dbl, "Avg.weighting"=w906:dbl[])  [unwired: 2 out]
        n602 = local read "Channels"() -> (w887:u8)
        n603 = Not Equal To 0?(x=w925) -> (x != 0?=w897:bool)
        "Overload" <- w897
        n604 = Unbundle By Name(w874) -> ("Weighting Curve"=w866:T1)
        n605 = Equal To 0?(x=w884) -> (x = 0?=w883:bool)
        n606 = call "CRYChannel separate buffer array.vi"("N channels"=w887, "Buffer array in"=w941) -> ("First right channel"=w885:i32[], "First left channel"=w886:i32[])  [unwired: 8 out]
        n607 = local read "Sampling rate"() -> (w867:u32)
        n608 = property on="Overload" class="Bool (strict)"("闪烁"=w897) -> ()  [unwired: 2 in, 2 out]
        n609 = Select(t=w886, s=w883, f=w885) -> (s? t:f=w924:i32[])
        n610 = Increment(x=w927) -> (x+1=w905:i32)
        n611 = case shown="2" w880 {
          tunnel: w879 -> [w994 w996]
          tunnel: [w994 w995] -> w878
          frame 0, Default {
          }
          frame 2 {
            n612 = Divide(x=w996, y=512.0 ("cal factor1")) -> (x/y=w995:dbl)
          }
        }
        n613 = local read "Apply Correction"() -> (w865:bool)
        n614 = Multiply(x=w924, y=w878) -> (x*y=w852:dbl[])
        n615 = call "CRYCalc Eq Wave.vi"("EQ Curve"=w866, "Fs"=w867, "Wave In"=w852) -> ("Wave Out"=w851:dbl[])  [unwired: 7 in, 1 out]
        n616 = call <vilib>:"AC & DC Estimator.vi"("Signal (V)"=w851) -> ("AC estimate (Vrms)"=w936:dbl, "DC estimate (V)"=w935:dbl)
        n617 = case shown="False" w865 {
          tunnel: [w989 w992] -> w850
          tunnel: w851 -> [w989 w991]
          frame False {
          }
          frame True {
            n618 = local read "Sampling rate"() -> (w993:u32)
            n619 = local read "Corr Curve"() -> (w990:T1)
            n620 = call "CRYCalc Eq Wave.vi"("EQ Curve"=w990, "Fs"=w993, "Wave In"=w991) -> ("Wave Out"=w992:dbl[])  [unwired: 7 in, 1 out]
          }
        }
        n621 = case shown="0, Default" "AC/DC" {
          tunnel: w936 -> [w1045 _]
          tunnel: w935 -> [_ w1046]
          tunnel: [w1045 w1046] -> w873
          frame 0, Default {
          }
          frame 1 {
          }
        }
        n622 = local read "Lin/Exp"() -> (w854:i32)
        n623 = Flatten To String(anything=w873) -> (data string=w915:string)  [unwired: 1 in, 4 out]
        n624 = Enqueue Element(queue=w931, element=w915, error in (no error)=w930) -> (queue out=w928:refnum<queue>, error out=w929:errorcluster)  [unwired: 2 out]
        n625 = Get Queue Status(queue=w928, return elements? (F)=TRUE ("return elements"), error in (no error)=w929) -> (queue out=w951:refnum<queue>, error out=w953:errorcluster, # elements in queue=w904:i32, elements=w926:string[])  [unwired: 4 out]
        n626 = Greater Or Equal?(x=w904, y=w876) -> (x >= y?=w877:bool)
        n627 = case "buffer full now?" shown="False" w877 {
          tunnel: w906 -> [w1023 w1025]
          tunnel: w904 -> [w1024 _]
          tunnel: [w1020 w1025] -> w933
          frame False {
            # "renormalize clipped\nweighting function"
            n628 = Array Subset(array=w1023, length=w1024) -> (w1022:dbl[])  [unwired: 1 in]
            n629 = Add Array Elements(numeric array=w1022) -> (sum=w1021:dbl)
            n630 = Divide(x=w1022, y=w1021) -> (x/y=w1020:dbl[])
          }
          frame True {
          }
        }
        n631 = for {
          tunnel: [w1044] -> w875 mode=indexing
          tunnel: w926 -> [w1043] mode=indexing
          n632 = Unflatten From String(type=0.0, binary string=w1043) -> (value=w1044:dbl)  [unwired: 1 in, 4 out]
        }
        n633 = case shown="1" w854 {
          tunnel: w868 -> [_ w972]
          tunnel: [_ w971] -> w863
          tunnel: w850 -> [w966 w968]
          tunnel: [w967 w969] -> w853
          tunnel: [w966 w968] -> w846
          frame 0, Default {
            n634 = call-poly <vilib>:"Mean.vi"("X"=w966) -> ("mean"=w967:dbl)  [unwired: 1 out]
          }
          frame 1 {
            w981 = 1.0 ("x")
            n635 = local read "Sampling rate"() -> (w979:u32)
            n636 = Multiply(x=w972, y=0.05 ("x")) -> (x*y=w976:dbl)
            n637 = Multiply(x=w976, y=w979) -> (x*y=w971:dbl)
            n638 = Increment(x=w971) -> (x+1=w978:dbl)
            n639 = Square(x=w968) -> (x^2=w975:dbl[])
            n640 = Divide(x=w981, y=w978) -> (x/y=w973:dbl)
            n641 = local read "y(n-1)"() -> (w980:dbl)
            n642 = Subtract(x=w981, y=w973) -> (x-y=w974:dbl)
            n643 = for {
              tunnel: w975 -> [w988] mode=indexing
              tunnel: w973 -> [w987]
              tunnel: w974 -> [w985]
              shift-right: [w982] -> _
              shift-left: w980 -> [w986]
              tunnel: [w982] -> w970
              tunnel: [w982] -> _ mode=indexing
              n644 = Multiply(x=w988, y=w987) -> (x*y=w984:dbl)
              n645 = Multiply(x=w986, y=w985) -> (x*y=w983:dbl)
              n646 = Add(x=w984, y=w983) -> (x+y=w982:dbl)
            }
            "y(n-1)" <- w970
            n647 = Square Root(x=w970) -> (sqrt(x)=w969:dbl)
          }
        }
        n648 = Absolute Value(x=w846) -> (abs(x)=w849:dbl[])
        n649 = Array Max & Min(array=w849) -> (max value=w848:dbl)  [unwired: 3 out]
        n650 = Array Max & Min(array=w849) -> (min value=w847:dbl)  [unwired: 3 out]
        n651 = call-poly <vilib>:"Dot Product.vi"("Y Vector"=w933, "X Vector"=w875) -> ()  [unwired: 2 out]
        n652 = Max & Min(x=w853, y=w912) -> (min(x,y)=w857:dbl)  [unwired: 1 out]
        n653 = Max & Min(x=w853, y=w862) -> (max(x,y)=w859:dbl)  [unwired: 1 out]
        n654 = Max & Min(x=w848, y=w911) -> (max(x,y)=w858:dbl)  [unwired: 1 out]
        n655 = Max & Min(x=w847, y=w861) -> (min(x,y)=w856:dbl)  [unwired: 1 out]
        n656 = disable-structure shown="Disabled" {
          disable-tunnel: w863 -> [w965 _]
          disable-tunnel: w851 -> [w956 _]
          disable-tunnel: w850 -> [w955 _]
          frame Disabled {
            w959 = 2400 ("index")
            n657 = local read "WWWW 2"() -> (w961:dbl[])
            n658 = local read "WWWW"() -> (w964:dbl[])
            n659 = Build Array (concatenate)(w964, w956) -> (w962:dbl[])
            n660 = Build Array (concatenate)(w961, w955) -> (w960:dbl[])
            n661 = Array Subset(array=w962, index=w959, length=w965) -> (w958:dbl[])
            "WWWW" <- w958
            n662 = Array Subset(array=w960, index=w959, length=w965) -> (w957:dbl[])
            "WWWW 2" <- w957
            n663 = Build Array(w958, w957) -> (→"Waveform Graph":dbl[][])
          }
          frame Enabled {
          }
        }
        n664 = local read "Mode"() -> (w910:i32)
        n665 = local read "Level"() -> (w860:i32)
        n666 = case shown="2" w910 {
          tunnel: [w1007 w1011 w1017] -> w855
          tunnel: w860 -> [_ w1010 w1016]
          tunnel: w859 -> [_ w1009 _]
          tunnel: w858 -> [_ w1008 _]
          tunnel: w853 -> [w1007 _ _]
          tunnel: w857 -> [_ _ w1015]
          tunnel: w856 -> [_ _ w1014]
          frame 0, Default {
          }
          frame 1 {
            n667 = case shown="1" w1010 {
              tunnel: [w1012 w1013] -> w1011
              tunnel: w1009 -> [w1012 _]
              tunnel: w1008 -> [_ w1013]
              frame 0, Default {
                # "RMS"
              }
              frame 1 {
                # "Peak"
              }
            }
          }
          frame 2 {
            n668 = case shown="1" w1016 {
              tunnel: [w1018 w1019] -> w1017
              tunnel: w1015 -> [w1018 _]
              tunnel: w1014 -> [_ w1019]
              frame 0, Default {
                # "RMS"
              }
              frame 1 {
                # "Peak"
              }
            }
          }
        }
        "InputLevel" <- w855
        n669 = local read "dB ref."() -> (w895:dbl)
        n670 = Divide(x=w855, y=w903) -> (x/y=w872:dbl)
        n671 = local read "unit"() -> (w894:string)
        n672 = Logarithm Base 10(1:w872) -> (0:w871:dbl)
        n673 = Bundle By Name(cluster=T2 {"InputLevel"=0.0, "unit"="", "dB ref."=0.0}, "InputLevel"=w855, "unit"=w894, "dB ref."=w895) -> (→"InputLevel Out":T2)
        n674 = Bundle By Name(cluster=w891, "avg. hold"=w853, "rms max"=w859, "rms min"=w857, "peak max"=w858, "peak min"=w856) -> (w920:T11)
        n675 = Multiply(x=w871, y=20.0) -> (x*y=w869:dbl)
        n676 = Bundle(w869, "cal factor3"=w899) -> (→"dB":cluster{dbl, "cal factor3":dbl})  [unwired: 1 out]
      }
    }
  }
  n677 = Unbundle By Name(w4) -> ("avg. complete"=w3:i32)
  n678 = Release Queue(queue=w11, error in (no error)=w10) -> (error out=w9:errorcluster)  [unwired: 3 out]
  n679 = call <vilib>:"Simple Error Handler.vi"("error in (no error)"=w9) -> ("error out"=w6:errorcluster)  [unwired: 1 in, 7 out]
  n680 = case shown="False" w5 {
    tunnel: [w1156 ""] -> w16
    frame False {
      n681 = call "CRYGet Error Message.vi"("Error No"=0, "Kind"="Multimeter") -> ("Message"=w1156:string)  [unwired: 4 in, 5 out]
      n682 = One Button Dialog(message=w1156) -> ()  [unwired: 2 out]
    }
    frame True {
    }
  }
  n683 = stacked-sequence {
    tunnel: w16 -> [_ _ _ _]
    tunnel: w6 -> [_ _ _ _]
    tunnel: w3 -> [_ w1181 _ _]
    frame #0 {
      w1164 = u32 0 ("nSampleFreq")
      n684 = local read "Rcv Idx"() -> (w1160:u16)
      n685 = local read "isMain"() -> (w1161:bool)
      n686 = call "CRYClear Main Receiver Array.vi"("isMain"=w1161, "Rcv Idx"=w1160) -> ()  [unwired: 10 in]
      n687 = local read "ASIO_Inited"() -> (w1162:bool)
      n688 = local read "Audio Driver"() -> (w1163:u16)
      n689 = local read "Device In"() -> (w1167:u32)
      n690 = local read "taskID"() -> (w1165:u32)
      n691 = case shown="2" w1163 {
        tunnel: w1162 -> [w1168 _]
        frame 2 {
          n692 = case shown="True" w1168 {
            frame False {
            }
            frame True {
              n693 = local read "Asio OCI"() -> (w1170:u32)
              n694 = local read "Channel In"() -> (w1169:u16)
              n695 = local write "ASIO_Inited"(FALSE ("ASIO_Inited")) -> ()
              n696 = call "CRYASIO Close Cur Channel & Dev.vi"("Limit"=w1170, "isInput?"=TRUE, "Channel Out"=w1169) -> ()  [unwired: 9 in]
            }
          }
        }
        frame 0, Default {
        }
      }
      n697 = dll-call lib="D:/A_CRYSoundLab_Work/CRY6181/CRYSound.dll" fn="GVContinueRecord"("DeviceID"=w1167, "nSampleFreq"=w1164, "nChannels"=w1164, "BitDepth"=w1164, "TimeRate"=w1164, "mode"=w1164, "nBufferUse"=w1164, "RealTime"=w1164, "timeOut"=w1164, "RecData"=i32[] [], "RecDataLen"=w1164, "OverHead"=w1164, "StartFlag"=w1164, "PauseFlag"=w1164, "ChangeFlag"=w1164, "taskID"=w1165) -> ()  [unwired: 9 in, 13 out]
    }
    frame #1 {
      # "?????????"
      n698 = local read "Apply Correction"() -> (w1187:bool)
      n699 = local read "Time Weighting"() -> (w1184:i32)
      n700 = local read "User Avg.Time(sec)"() -> (w1180:dbl)
      n701 = property on="Signal Path" class="Ring (strict)"() -> ("RingText.Text"=w1183:string)  [unwired: 2 in, 2 out]
      n702 = property on="Weighting" class="Ring (strict)"() -> ("RingText.Text"=w1188:string)  [unwired: 2 in, 2 out]
      n703 = local read "Channel In"() -> (w1190:u16)
      n704 = local read "Time(sec)"() -> (w1185:dbl)
      "Record time out" <- w1185
      n705 = local read "Lin/Exp"() -> (w1186:i32)
      n706 = global read "CRYMisc vis settings global.vi" "Rcv Index Array"() -> (w1175:T13)
      n707 = local read "Mode"() -> (w1189:i32)
      n708 = local read "Level"() -> (w1182:i32)
      n709 = local read "Cancel"() -> (w1179:bool)
      n710 = local read "Rcv Idx"() -> (w1173:u16)
      n711 = for {
        tunnel: w1175 -> [w1194] mode=indexing
        tunnel: [w1193] -> w1174 mode=indexing
        n712 = Unbundle By Name(w1194) -> ("Rcv Idx"=w1193:i32)
      }
      n713 = local write "Canceled?"(w1179) -> ()
      n714 = global read "CRYMisc vis settings global.vi" "Voltmeter Settings"() -> (w1178:T8)
      n715 = Bundle By Name(cluster=w1178, "Ave/Max/Min"=w1189, "Level"=w1182, "Channel"=w1190, "Signal Type"=w1183, "Weighting"=w1188, "Applay Correction"=w1187, "lin/exp avg"=w1186, "rec time (sec)"=w1185, "Time Weighting"=w1184, "Average Time (Sec)"=w1180) -> (w1192:T8)
      n716 = Search 1D Array(1D array=w1174, element=w1173) -> (index of element=w1177:i32)  [unwired: 1 in]
      n717 = Delete From Array(array=w1175, index=w1177) -> (array with subset deleted=w1176:T13)  [unwired: 1 in, 1 out]
      n718 = case shown="False" w1179 {
        tunnel: w1192 -> [w1195 _]
        frame False {
          n719 = flat-sequence {
            tunnel: w1195 -> [w1196]
            frame #0 {
              n720 = global write "CRYMisc vis settings global.vi" "Voltmeter Settings"(w1196) -> ()
            }
            frame #1 {
              n721 = local read "Manual"() -> (w1197:bool)
              n722 = case shown="False" w1197 {
                frame False {
                  n723 = call "CRYSave Virtual Data.vi"() -> ()  [unwired: 11 in, 1 out]
                }
                frame True {
                }
              }
            }
          }
        }
        frame True {
        }
      }
      n724 = call "CRYFlatten Multimeter.vi"("Voltmeter Settings"=w1192) -> ("Flat Voltmeter setup"=→"multimeter setup Out":string)  [unwired: 10 out]
      n725 = global write "CRYMisc vis settings global.vi" "Rcv Index Array"(w1176) -> ()
      "Averages out" <- w1181
    }
    frame #2 {
      w1202 = FALSE ("OK")
      n726 = global read "CRYMisc vis settings global.vi" "CloseAll Event"() -> (w1201:bool)
      n727 = local read "Menu"() -> (w1199:bool)
      n728 = Not(x=w1201) -> (.not. x?=w1200:bool)
      n729 = And(x=w1199, y=w1200) -> (x .and. y?=w1198:bool)
      n730 = case shown="True" w1198 {
        frame False {
        }
        frame True {
          n731 = local read "VI nID"() -> (w1204:i32)
          n732 = call "CRYOperator Process.vi"("VI ID"=w1204, "sAction"="Close", "sOperator Type"="OPERATOR_MULTIMETER" ("sAction")) -> ()  [unwired: 8 in, 1 out]
        }
      }
      n733 = local write "Cancel"(w1202) -> ()
      n734 = local write "OK"(w1202) -> ()
      n735 = case shown="True" "close at end" {
        frame False {
        }
        frame True {
          n736 = property class="VI"("前面板窗口:打开"=FALSE ("Front Panel Window:Open")) -> ()  [unwired: 2 in, 2 out]
        }
      }
    }
    frame #3 {
      n737 = local write "StateOut"(TRUE ("StateOut")) -> ()
    }
  }
